vi "PIV_Stats.vi"(0 "Data Folder":path=path "T:/Ensight_Data/NACA0015/NACA0015_NM_B/Test_A", 1 "PIV Meas Plane":enum16{"XY", "YZ", "XZ"}(ring)=enum."XZ", 2 "Row number":i32=1, 5 "Output Directory":path=path "T:/Ensight_Data/NACA0015/NACA0015_NM_B", 7 "XYZ Translation":dbl[](array[numeric])=[200.0, 8.0, -30.0], 9 "Case Name":string="Test_A_Case", 11 "PIV Freq (Hz)":dbl=7.25, 12 "Invert U":bool=TRUE, 13 "Invert V":bool) -> (4 "Progress Bar":i32(slide) scale=0.0..100.0, 6 "Status":string, 10 "# total vectors":i32=9858, 15 "# vectors without records":i16)   [LabVIEW 2011]
uses:
  <vilib>/Utility/error.llb/DialogType.ctl
  <vilib>/Analysis/1siggen.llb/Ramp Pattern by Samples.vi
  <vilib>/Analysis/NI_AALBase.lvlib
panel:
  out "VectRawData(time,spot)":dbl[][][](array[numeric])
  out "Position Array":dbl[][](array[numeric])
  out "Data Array":dbl[][][](array[numeric])
  out "Tmax":dbl=0.41379310344827586
  out "Max Record Length":i32=3
  out "Variable Names":string[](array[string])=["Record_Length", "CHC", "u_ms", "v_ms", "time_s", "Vel_mag_ms", "Turb_Stats_U_ms", "Turb_Stats_u2_m2s2", "Turb_Stats_u3_m3s3", "Turb_Stats_u4_m4s4", "Turb_Stats_TurbU_%", "Turb_Stats_Skew_u", "Turb_Stats_Kurt_u", "Turb_Stats_V_ms", "Turb_Stats_v2_m2s2", "Turb_Stats_v3_m3s3", "Turb_Stats_v4_m4s4", "Turb_Stats_TurbV_%", "Turb_Stats_Skew_v", "Turb_Stats_Kurt_v", "Turb_Stats_u2v2_m4s4", "Turb_Stats_uv3_m4s4", "Turb_Stats_u3v_m4s4", "Turb_Stats_uv2_m3s3", "Turb_Stats_u2v_m3s3", "Turb_Stats_uv_cc", "Turb_Stats_uv", "Turb_Stats_TKE_J", "Turb_Stats_Error_U_ms", "Turb_Stats_Error_u2_m2s2", "Turb_Stats_Error_u3_m3s3", "Turb_Stats_Error_u4_m4s4", "Turb_Stats_Error_TurbU_%", "Turb_Stats_Error_Skew_u", "Turb_Stats_Error_Kurt_u", "Turb_Stats_Error_V_ms", "Turb_Stats_Error_v2_m2s2", "Turb_Stats_Error_v3_m3s3", "Turb_Stats_Error_v4_m4s4", "Turb_Stats_Error_TurbV_%", "Turb_Stats_Error_Skew_v", "Turb_Stats_Error_Kurt_v", "Turb_Stats_Error_u2v2_m4s4", "Turb_Stats_Error_uv3_m4s4", "Turb_Stats_Error_u3v_m4s4", "Turb_Stats_Error_uv2_m3s3", "Turb_Stats_Error_u2v_m3s3", "Turb_Stats_Error_uv_cc", "Turb_Stats_Error_uv", "Turb_Stats_Error_TKE_J"]
  out "File Paths":path[][](array[path])=[[path "C:/Users/Nick/Desktop/Test/Testing/ENSI_0000.case", path "C:/Users/Nick/Desktop/Test/Testing/ENSI_0000.geo", path "C:/Users/Nick/Desktop/Test/Testing/ENSI_0000.var1", path "C:/Users/Nick/Desktop/Test/Testing/ENSI_0000.var2", path "C:/Users/Nick/Desktop/Test/Testing/ENSI_0000.var3", path "C:/Users/Nick/Desktop/Test/Testing/ENSI_0000.var4", path "C:/Users/Nick/Desktop/Test/Testing/ENSI_0000.var5", path "C:/Users/Nick/Desktop/Test/Testing/ENSI_0000.var6", path "C:/Users/Nick/Desktop/Test/Testing/ENSI_0000.var7", path "C:/Users/Nick/Desktop/Test/Testing/ENSI_0000.var8", path "C:/Users/Nick/Desktop/Test/Testing/ENSI_0000.var9", path "C:/Users/Nick/Desktop/Test/Testing/ENSI_0000.var10", path "C:/Users/Nick/Desktop/Test/Testing/ENSI_0000.var11", path "C:/Users/Nick/Desktop/Test/Testing/ENSI_0000.var12", path "C:/Users/Nick/Desktop/Test/Testing/ENSI_0000.var13", path "C:/Users/Nick/Desktop/Test/Testing/ENSI_0000.var14", path "C:/Users/Nick/Desktop/Test/Testing/ENSI_0000.var15", path "C:/Users/Nick/Desktop/Test/Testing/ENSI_0000.var16", path "C:/Users/Nick/Desktop/Test/Testing/ENSI_0000.var17", path "C:/Users/Nick/Desktop/Test/Testing/ENSI_0000.var18", path "C:/Users/Nick/Desktop/Test/Testing/ENSI_0000.var19", path "C:/Users/Nick/Desktop/Test/Testing/ENSI_0000.var20", path "C:/Users/Nick/Desktop/Test/Testing/ENSI_0000.var21", path "C:/Users/Nick/Desktop/Test/Testing/ENSI_0000.var22", path "C:/Users/Nick/Desktop/Test/Testing/ENSI_0000.var23", path "C:/Users/Nick/Desktop/Test/Testing/ENSI_0000.var24", path "C:/Users/Nick/Desktop/Test/Testing/ENSI_0000.var25", path "C:/Users/Nick/Desktop/Test/Testing/ENSI_0000.var26", path "C:/Users/Nick/Desktop/Test/Testing/ENSI_0000.var27", path "C:/Users/Nick/Desktop/Test/Testing/ENSI_0000.var28", path "C:/Users/Nick/Desktop/Test/Testing/ENSI_0000.var29", path "C:/Users/Nick/Desktop/Test/Testing/ENSI_0000.var30", path "C:/Users/Nick/Desktop/Test/Testing/ENSI_0000.var31", path "C:/Users/Nick/Desktop/Test/Testing/ENSI_0000.var32", path "C:/Users/Nick/Desktop/Test/Testing/ENSI_0000.var33", path "C:/Users/Nick/Desktop/Test/Testing/ENSI_0000.var34", path "C:/Users/Nick/Desktop/Test/Testing/ENSI_0000.var35", path "C:/Users/Nick/Desktop/Test/Testing/ENSI_0000.var36", path "C:/Users/Nick/Desktop/Test/Testing/ENSI_0000.var37", path "C:/Users/Nick/Desktop/Test/Testing/ENSI_0000.var38", path "C:/Users/Nick/Desktop/Test/Testing/ENSI_0000.var39", path "C:/Users/Nick/Desktop/Test/Testing/ENSI_0000.var40", path "C:/Users/Nick/Desktop/Test/Testing/ENSI_0000.var41", path "C:/Users/Nick/Desktop/Test/Testing/ENSI_0000.var42", path "C:/Users/Nick/Desktop/Test/Testing/ENSI_0000.var43", path "C:/Users/Nick/Desktop/Test/Testing/ENSI_0000.var44", path "C:/Users/Nick/Desktop/Test/Testing/ENSI_0000.var45", path "C:/Users/Nick/Desktop/Test/Testing/ENSI_0000.var46", path "C:/Users/Nick/Desktop/Test/Testing/ENSI_0000.var47", path "C:/Users/Nick/Desktop/Test/Testing/ENSI_0000.var48", path "C:/Users/Nick/Desktop/Test/Testing/ENSI_0000.var49", path "C:/Users/Nick/Desktop/Test/Testing/ENSI_0000.var50"], [path "C:/Users/Nick/Desktop/Test/Testing/ENSI_0001.case", path "C:/Users/Nick/Desktop/Test/Testing/ENSI_0001.geo", path "C:/Users/Nick/Desktop/Test/Testing/ENSI_0001.var1", path "C:/Users/Nick/Desktop/Test/Testing/ENSI_0001.var2", path "C:/Users/Nick/Desktop/Test/Testing/ENSI_0001.var3", path "C:/Users/Nick/Desktop/Test/Testing/ENSI_0001.var4", path "C:/Users/Nick/Desktop/Test/Testing/ENSI_0001.var5", path "C:/Users/Nick/Desktop/Test/Testing/ENSI_0001.var6", path "C:/Users/Nick/Desktop/Test/Testing/ENSI_0001.var7", path "C:/Users/Nick/Desktop/Test/Testing/ENSI_0001.var8", path "C:/Users/Nick/Desktop/Test/Testing/ENSI_0001.var9", path "C:/Users/Nick/Desktop/Test/Testing/ENSI_0001.var10", path "C:/Users/Nick/Desktop/Test/Testing/ENSI_0001.var11", path "C:/Users/Nick/Desktop/Test/Testing/ENSI_0001.var12", path "C:/Users/Nick/Desktop/Test/Testing/ENSI_0001.var13", path "C:/Users/Nick/Desktop/Test/Testing/ENSI_0001.var14", path "C:/Users/Nick/Desktop/Test/Testing/ENSI_0001.var15", path "C:/Users/Nick/Desktop/Test/Testing/ENSI_0001.var16", path "C:/Users/Nick/Desktop/Test/Testing/ENSI_0001.var17", path "C:/Users/Nick/Desktop/Test/Testing/ENSI_0001.var18", path "C:/Users/Nick/Desktop/Test/Testing/ENSI_0001.var19", path "C:/Users/Nick/Desktop/Test/Testing/ENSI_0001.var20", path "C:/Users/Nick/Desktop/Test/Testing/ENSI_0001.var21", path "C:/Users/Nick/Desktop/Test/Testing/ENSI_0001.var22", path "C:/Users/Nick/Desktop/Test/Testing/ENSI_0001.var23", path "C:/Users/Nick/Desktop/Test/Testing/ENSI_0001.var24", path "C:/Users/Nick/Desktop/Test/Testing/ENSI_0001.var25", path "C:/Users/Nick/Desktop/Test/Testing/ENSI_0001.var26", path "C:/Users/Nick/Desktop/Test/Testing/ENSI_0001.var27", path "C:/Users/Nick/Desktop/Test/Testing/ENSI_0001.var28", path "C:/Users/Nick/Desktop/Test/Testing/ENSI_0001.var29", path "C:/Users/Nick/Desktop/Test/Testing/ENSI_0001.var30", path "C:/Users/Nick/Desktop/Test/Testing/ENSI_0001.var31", path "C:/Users/Nick/Desktop/Test/Testing/ENSI_0001.var32", path "C:/Users/Nick/Desktop/Test/Testing/ENSI_0001.var33", path "C:/Users/Nick/Desktop/Test/Testing/ENSI_0001.var34", path "C:/Users/Nick/Desktop/Test/Testing/ENSI_0001.var35", path "C:/Users/Nick/Desktop/Test/Testing/ENSI_0001.var36", path "C:/Users/Nick/Desktop/Test/Testing/ENSI_0001.var37", path "C:/Users/Nick/Desktop/Test/Testing/ENSI_0001.var38", path "C:/Users/Nick/Desktop/Test/Testing/ENSI_0001.var39", path "C:/Users/Nick/Desktop/Test/Testing/ENSI_0001.var40", path "C:/Users/Nick/Desktop/Test/Testing/ENSI_0001.var41", path "C:/Users/Nick/Desktop/Test/Testing/ENSI_0001.var42", path "C:/Users/Nick/Desktop/Test/Testing/ENSI_0001.var43", path "C:/Users/Nick/Desktop/Test/Testing/ENSI_0001.var44", path "C:/Users/Nick/Desktop/Test/Testing/ENSI_0001.var45", path "C:/Users/Nick/Desktop/Test/Testing/ENSI_0001.var46", path "C:/Users/Nick/Desktop/Test/Testing/ENSI_0001.var47", path "C:/Users/Nick/Desktop/Test/Testing/ENSI_0001.var48", path "C:/Users/Nick/Desktop/Test/Testing/ENSI_0001.var49", path "C:/Users/Nick/Desktop/Test/Testing/ENSI_0001.var50"], [path "C:/Users/Nick/Desktop/Test/Testing/ENSI_0002.case", path "C:/Users/Nick/Desktop/Test/Testing/ENSI_0002.geo", path "C:/Users/Nick/Desktop/Test/Testing/ENSI_0002.var1", path "C:/Users/Nick/Desktop/Test/Testing/ENSI_0002.var2", path "C:/Users/Nick/Desktop/Test/Testing/ENSI_0002.var3", path "C:/Users/Nick/Desktop/Test/Testing/ENSI_0002.var4", path "C:/Users/Nick/Desktop/Test/Testing/ENSI_0002.var5", path "C:/Users/Nick/Desktop/Test/Testing/ENSI_0002.var6", path "C:/Users/Nick/Desktop/Test/Testing/ENSI_0002.var7", path "C:/Users/Nick/Desktop/Test/Testing/ENSI_0002.var8", path "C:/Users/Nick/Desktop/Test/Testing/ENSI_0002.var9", path "C:/Users/Nick/Desktop/Test/Testing/ENSI_0002.var10", path "C:/Users/Nick/Desktop/Test/Testing/ENSI_0002.var11", path "C:/Users/Nick/Desktop/Test/Testing/ENSI_0002.var12", path "C:/Users/Nick/Desktop/Test/Testing/ENSI_0002.var13", path "C:/Users/Nick/Desktop/Test/Testing/ENSI_0002.var14", path "C:/Users/Nick/Desktop/Test/Testing/ENSI_0002.var15", path "C:/Users/Nick/Desktop/Test/Testing/ENSI_0002.var16", path "C:/Users/Nick/Desktop/Test/Testing/ENSI_0002.var17", path "C:/Users/Nick/Desktop/Test/Testing/ENSI_0002.var18", path "C:/Users/Nick/Desktop/Test/Testing/ENSI_0002.var19", path "C:/Users/Nick/Desktop/Test/Testing/ENSI_0002.var20", path "C:/Users/Nick/Desktop/Test/Testing/ENSI_0002.var21", path "C:/Users/Nick/Desktop/Test/Testing/ENSI_0002.var22", path "C:/Users/Nick/Desktop/Test/Testing/ENSI_0002.var23", path "C:/Users/Nick/Desktop/Test/Testing/ENSI_0002.var24", path "C:/Users/Nick/Desktop/Test/Testing/ENSI_0002.var25", path "C:/Users/Nick/Desktop/Test/Testing/ENSI_0002.var26", path "C:/Users/Nick/Desktop/Test/Testing/ENSI_0002.var27", path "C:/Users/Nick/Desktop/Test/Testing/ENSI_0002.var28", path "C:/Users/Nick/Desktop/Test/Testing/ENSI_0002.var29", path "C:/Users/Nick/Desktop/Test/Testing/ENSI_0002.var30", path "C:/Users/Nick/Desktop/Test/Testing/ENSI_0002.var31", path "C:/Users/Nick/Desktop/Test/Testing/ENSI_0002.var32", path "C:/Users/Nick/Desktop/Test/Testing/ENSI_0002.var33", path "C:/Users/Nick/Desktop/Test/Testing/ENSI_0002.var34", path "C:/Users/Nick/Desktop/Test/Testing/ENSI_0002.var35", path "C:/Users/Nick/Desktop/Test/Testing/ENSI_0002.var36", path "C:/Users/Nick/Desktop/Test/Testing/ENSI_0002.var37", path "C:/Users/Nick/Desktop/Test/Testing/ENSI_0002.var38", path "C:/Users/Nick/Desktop/Test/Testing/ENSI_0002.var39", path "C:/Users/Nick/Desktop/Test/Testing/ENSI_0002.var40", path "C:/Users/Nick/Desktop/Test/Testing/ENSI_0002.var41", path "C:/Users/Nick/Desktop/Test/Testing/ENSI_0002.var42", path "C:/Users/Nick/Desktop/Test/Testing/ENSI_0002.var43", path "C:/Users/Nick/Desktop/Test/Testing/ENSI_0002.var44", path "C:/Users/Nick/Desktop/Test/Testing/ENSI_0002.var45", path "C:/Users/Nick/Desktop/Test/Testing/ENSI_0002.var46", path "C:/Users/Nick/Desktop/Test/Testing/ENSI_0002.var47", path "C:/Users/Nick/Desktop/Test/Testing/ENSI_0002.var48", path "C:/Users/Nick/Desktop/Test/Testing/ENSI_0002.var49", path "C:/Users/Nick/Desktop/Test/Testing/ENSI_0002.var50"]]
  out "ALL filepath":path=path "C:/Users/Nick/Desktop/Test/Testing/ENSI_all.case"
  out "time s":dbl[](array[numeric])=[0.0, 0.20689655172413793, 0.41379310344827586]
  out "File Array":path[](array[path])=[path "T:/Ensight_Data/NACA0015/NACA0015_NM_A/Test_A_Trans/New folder/Test_A000000.T076.D000.P000.H000.L.vec", path "T:/Ensight_Data/NACA0015/NACA0015_NM_A/Test_A_Trans/New folder/Test_A000001.T076.D000.P000.H000.L.vec", path "T:/Ensight_Data/NACA0015/NACA0015_NM_A/Test_A_Trans/New folder/Test_A000002.T076.D000.P000.H000.L.vec"]
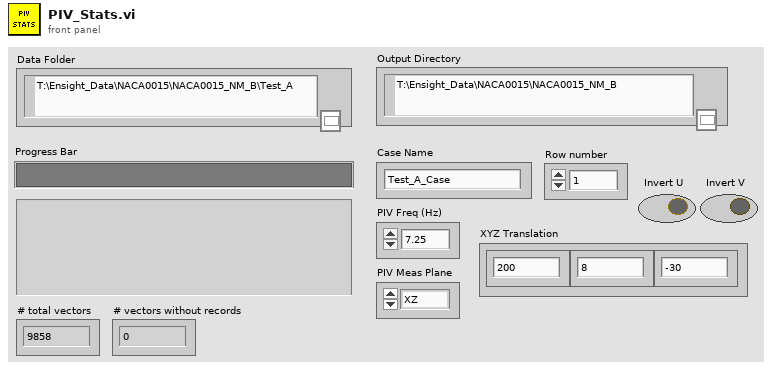
[diagram p1: front panel]
types:
  T1 = cluster{"Record Length":dbl, "CHC":dbl[], "u m/s":dbl[], "v m/s":dbl[], "time s":dbl[], "Vel mag m/s":dbl[], "XYZ Position":dbl[], " Turb Stats":cluster{"U m/s":dbl, "u2 m2/s2":dbl, "u3 m3/s3":dbl, "u4 m4/s4":dbl, "TurbU %":dbl, "Skew_u":dbl, "Kurt_u":dbl, "V m/s":dbl, "v2 m2/s2":dbl, "v3 m3/s3":dbl, "v4 m4/s4":dbl, "TurbV %":dbl, "Skew_v":dbl, "Kurt_v":dbl, "u2v2 m4/s4":dbl, "uv3 m4/s4":dbl, "u3v m4/s4":dbl, "uv2 m3/s3":dbl, "u2v m3/s3":dbl, "uv_cc":dbl, "uv":dbl, "TKE J":dbl}[], "Turb Stats Error":cluster{"U m/s":dbl, "u2 m2/s2":dbl, "u3 m3/s3":dbl, "u4 m4/s4":dbl, "TurbU %":dbl, "Skew_u":dbl, "Kurt_u":dbl, "V m/s":dbl, "v2 m2/s2":dbl, "v3 m3/s3":dbl, "v4 m4/s4":dbl, "TurbV %":dbl, "Skew_v":dbl, "Kurt_v":dbl, "u2v2 m4/s4":dbl, "uv3 m4/s4":dbl, "u3v m4/s4":dbl, "uv2 m3/s3":dbl, "u2v m3/s3":dbl, "uv_cc":dbl, "uv":dbl, "TKE J":dbl}[], "u (good)":dbl[], "v (good)":dbl[]}
  T2 = cluster{"Record Length":dbl, "CHC":dbl[], "u m/s":dbl[], "v m/s":dbl[], "time s":dbl[], "Vel mag m/s":dbl[], "XYZ Position":dbl[], " Turb Stats":cluster{"U m/s":dbl, "u2 m2/s2":dbl, "u3 m3/s3":dbl, "u4 m4/s4":dbl, "TurbU %":dbl, "Skew_u":dbl, "Kurt_u":dbl, "V m/s":dbl, "v2 m2/s2":dbl, "v3 m3/s3":dbl, "v4 m4/s4":dbl, "TurbV %":dbl, "Skew_v":dbl, "Kurt_v":dbl, "u2v2 m4/s4":dbl, "uv3 m4/s4":dbl, "u3v m4/s4":dbl, "uv2 m3/s3":dbl, "u2v m3/s3":dbl, "uv_cc":dbl, "uv":dbl, "TKE J":dbl}[], "Turb Stats Error":cluster{"U m/s":dbl, "u2 m2/s2":dbl, "u3 m3/s3":dbl, "u4 m4/s4":dbl, "TurbU %":dbl, "Skew_u":dbl, "Kurt_u":dbl, "V m/s":dbl, "v2 m2/s2":dbl, "v3 m3/s3":dbl, "v4 m4/s4":dbl, "TurbV %":dbl, "Skew_v":dbl, "Kurt_v":dbl, "u2v2 m4/s4":dbl, "uv3 m4/s4":dbl, "u3v m4/s4":dbl, "uv2 m3/s3":dbl, "u2v m3/s3":dbl, "uv_cc":dbl, "uv":dbl, "TKE J":dbl}[], "u (good)":dbl[], "v (good)":dbl[]}[]
  T3 = cluster{"U m/s":dbl, "u2 m2/s2":dbl, "u3 m3/s3":dbl, "u4 m4/s4":dbl, "TurbU %":dbl, "Skew_u":dbl, "Kurt_u":dbl, "V m/s":dbl, "v2 m2/s2":dbl, "v3 m3/s3":dbl, "v4 m4/s4":dbl, "TurbV %":dbl, "Skew_v":dbl, "Kurt_v":dbl, "u2v2 m4/s4":dbl, "uv3 m4/s4":dbl, "u3v m4/s4":dbl, "uv2 m3/s3":dbl, "u2v m3/s3":dbl, "uv_cc":dbl, "uv":dbl, "TKE J":dbl}
  T4 = cluster{"U m/s":dbl, "u2 m2/s2":dbl, "u3 m3/s3":dbl, "u4 m4/s4":dbl, "TurbU %":dbl, "Skew_u":dbl, "Kurt_u":dbl, "V m/s":dbl, "v2 m2/s2":dbl, "v3 m3/s3":dbl, "v4 m4/s4":dbl, "TurbV %":dbl, "Skew_v":dbl, "Kurt_v":dbl, "u2v2 m4/s4":dbl, "uv3 m4/s4":dbl, "u3v m4/s4":dbl, "uv2 m3/s3":dbl, "u2v m3/s3":dbl, "uv_cc":dbl, "uv":dbl, "TKE J":dbl}[]
  T5 = typedef "DialogType.ctl" = u16
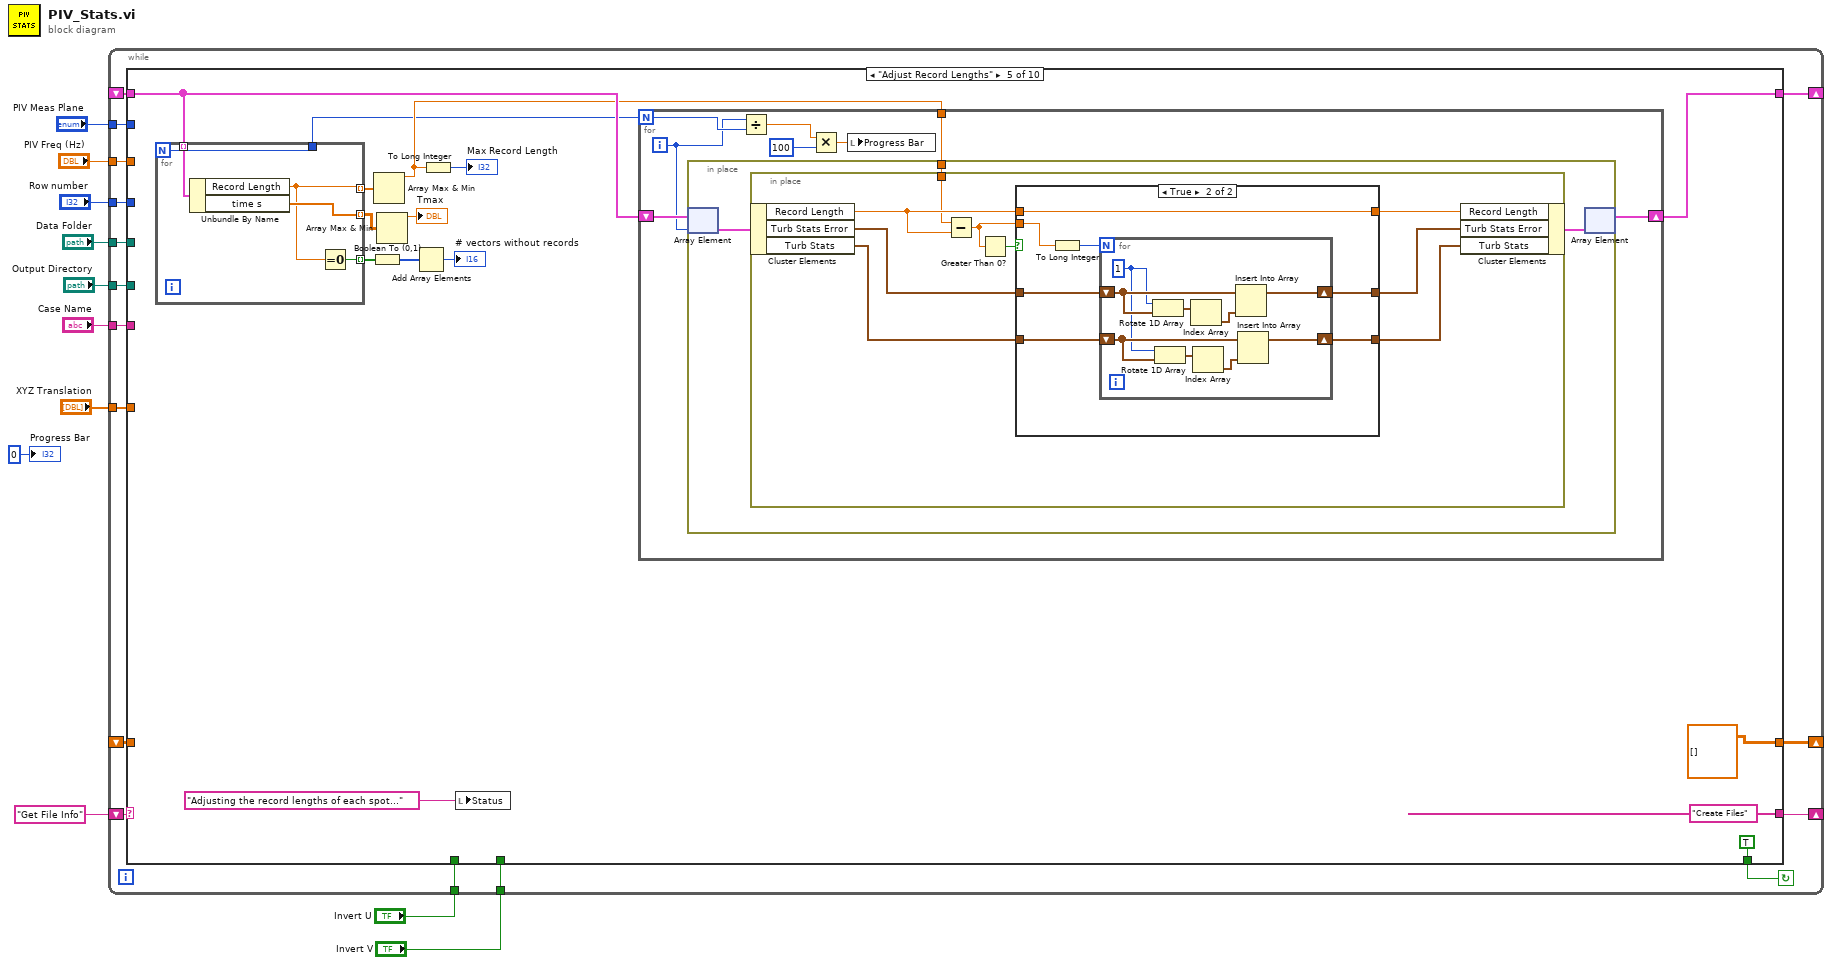
[diagram p0: block diagram]
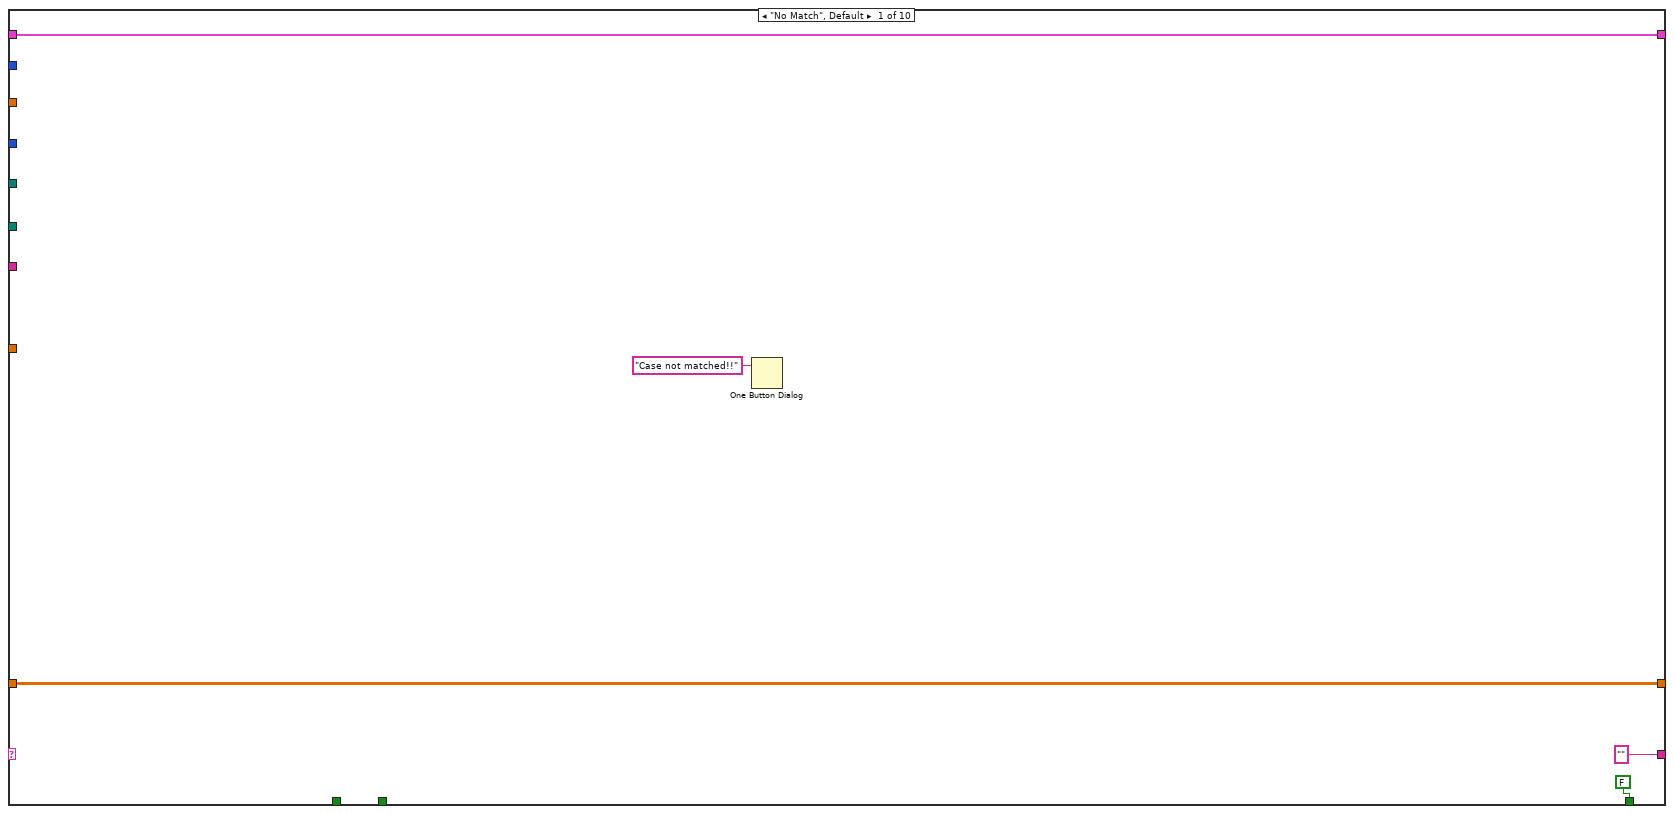
[diagram p2: hidden frame]
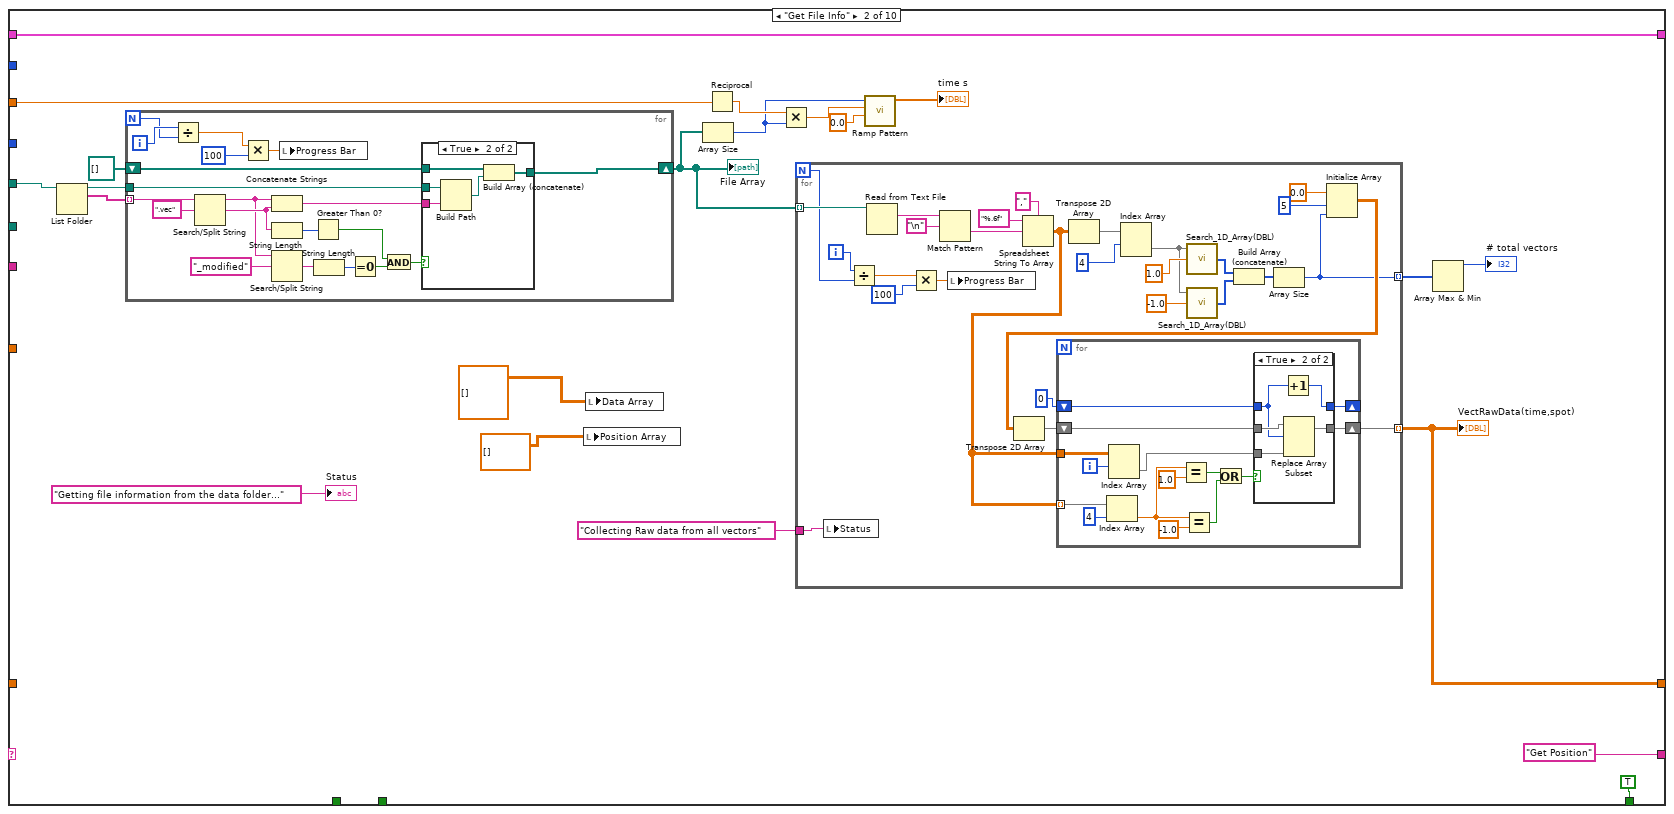
[diagram p3: hidden frame]
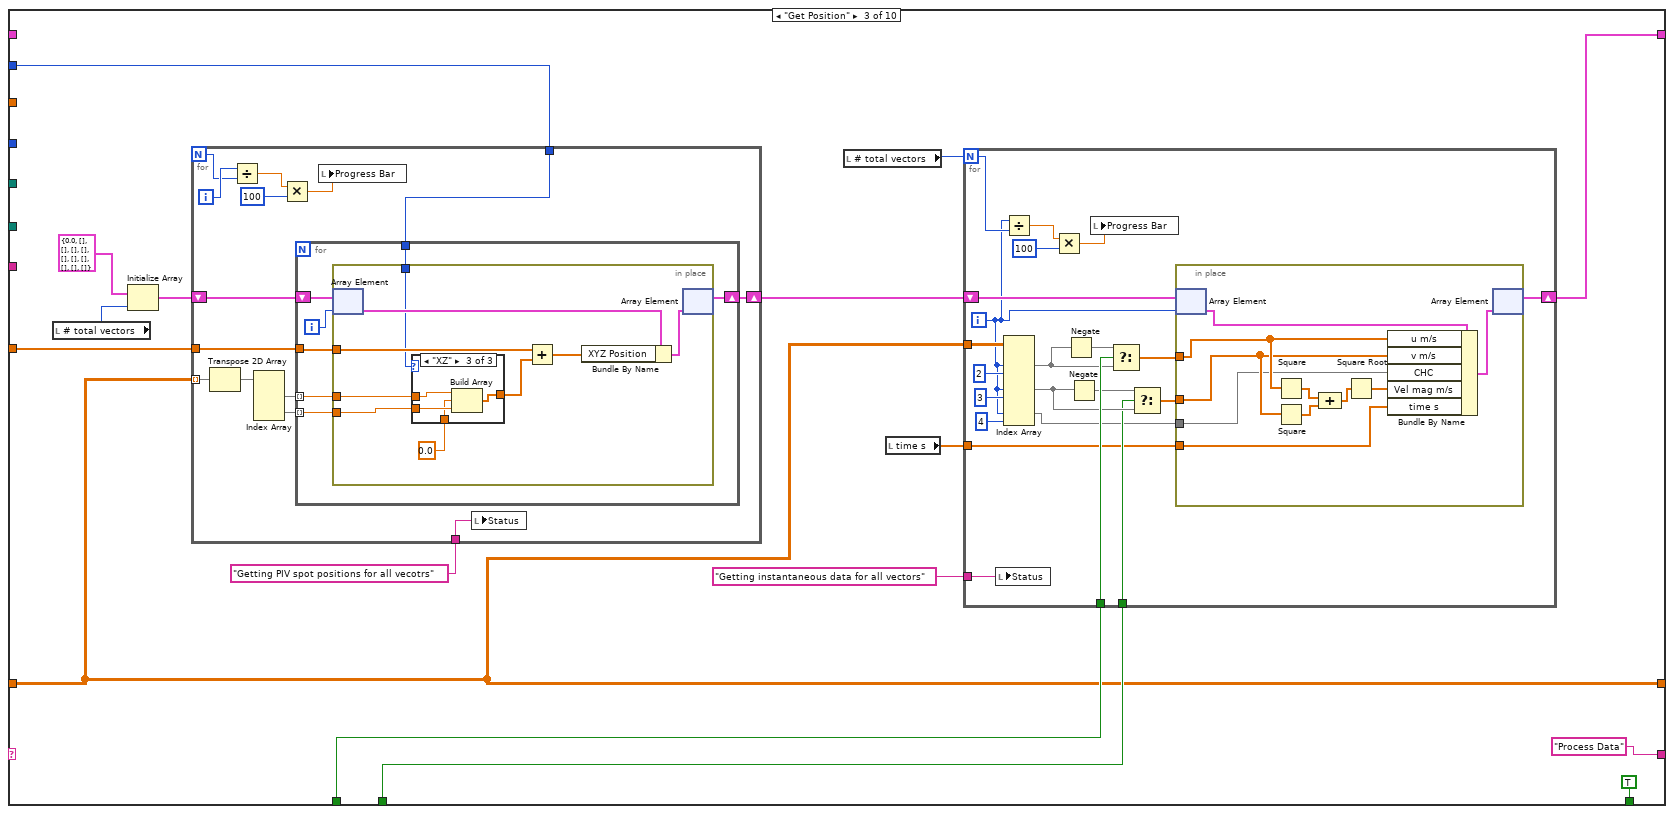
[diagram p6: hidden frame]
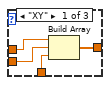
[diagram p7: hidden frame]
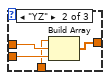
[diagram p8: hidden frame]
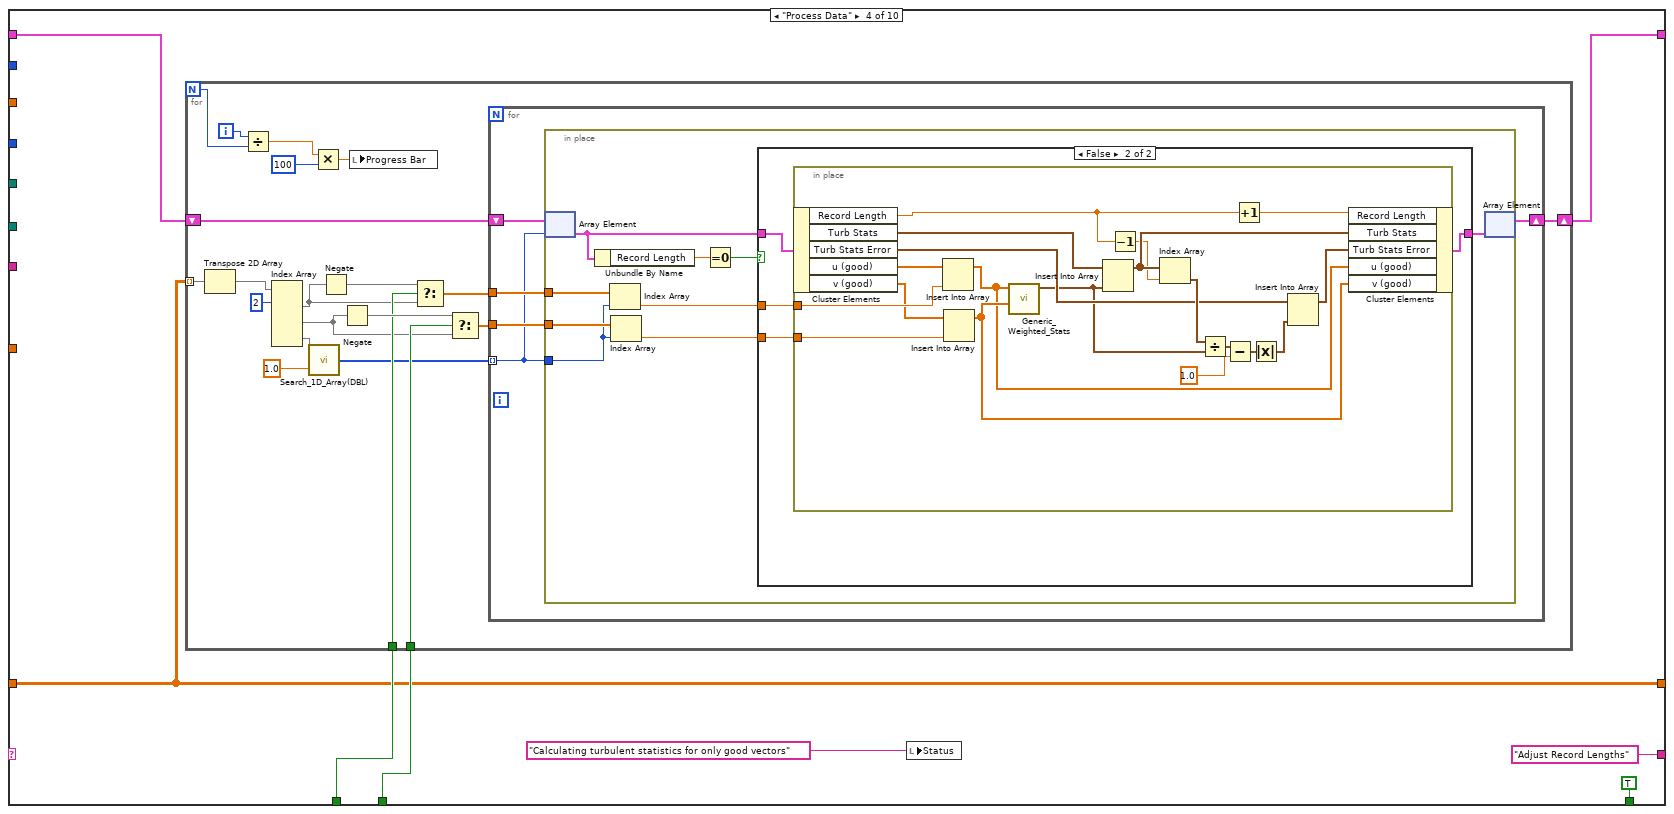
[diagram p9: hidden frame]
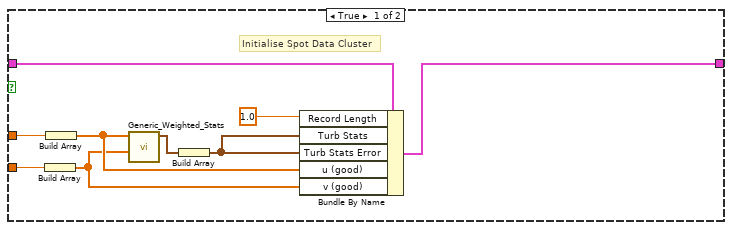
[diagram p10: hidden frame]
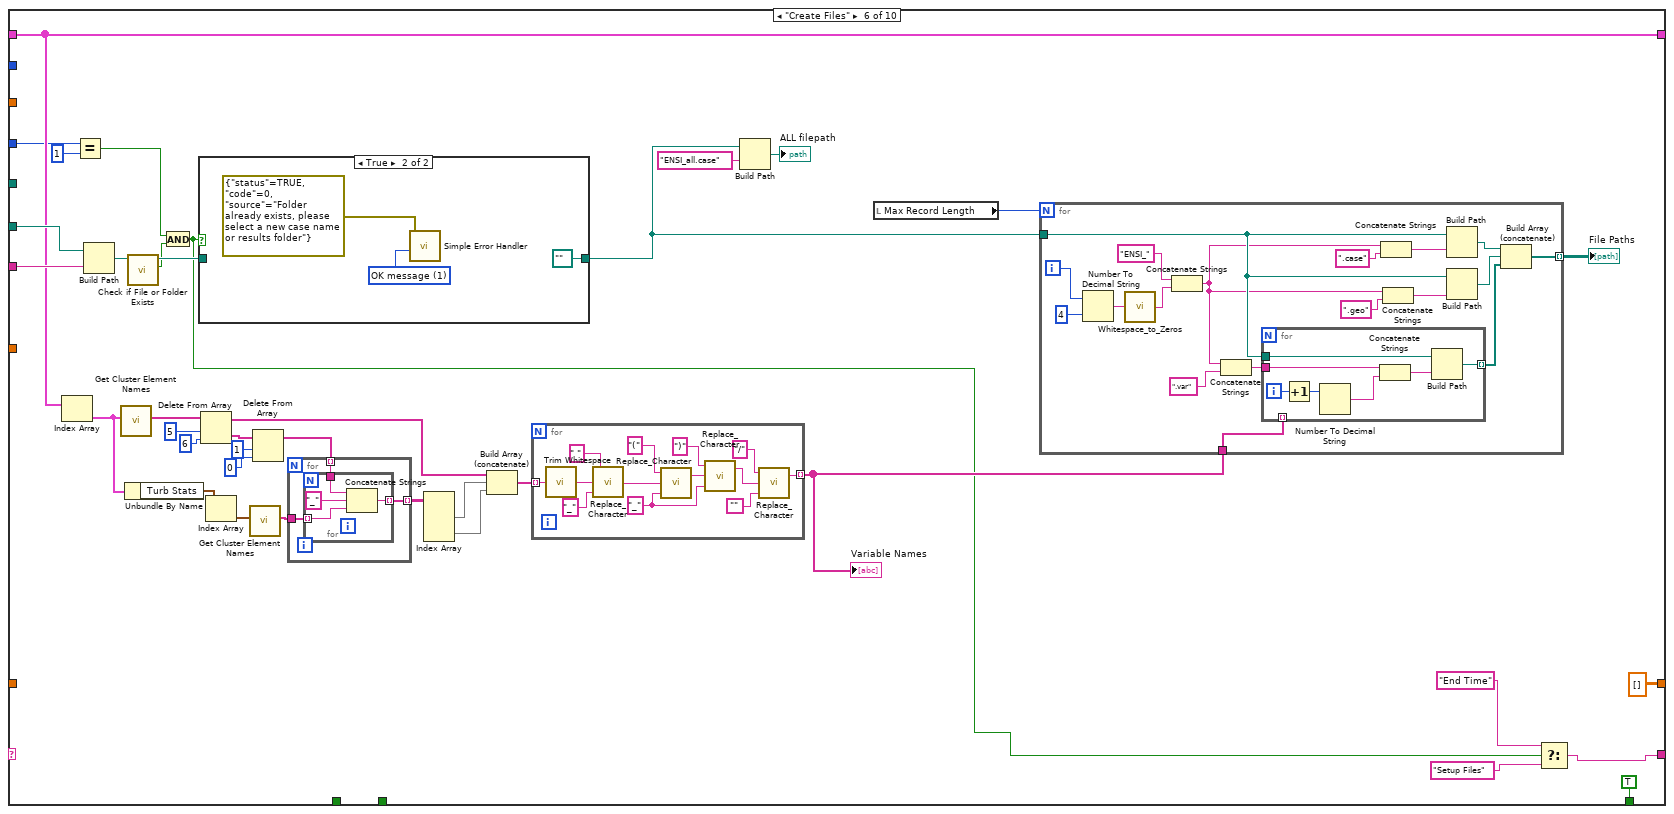
[diagram p12: hidden frame]
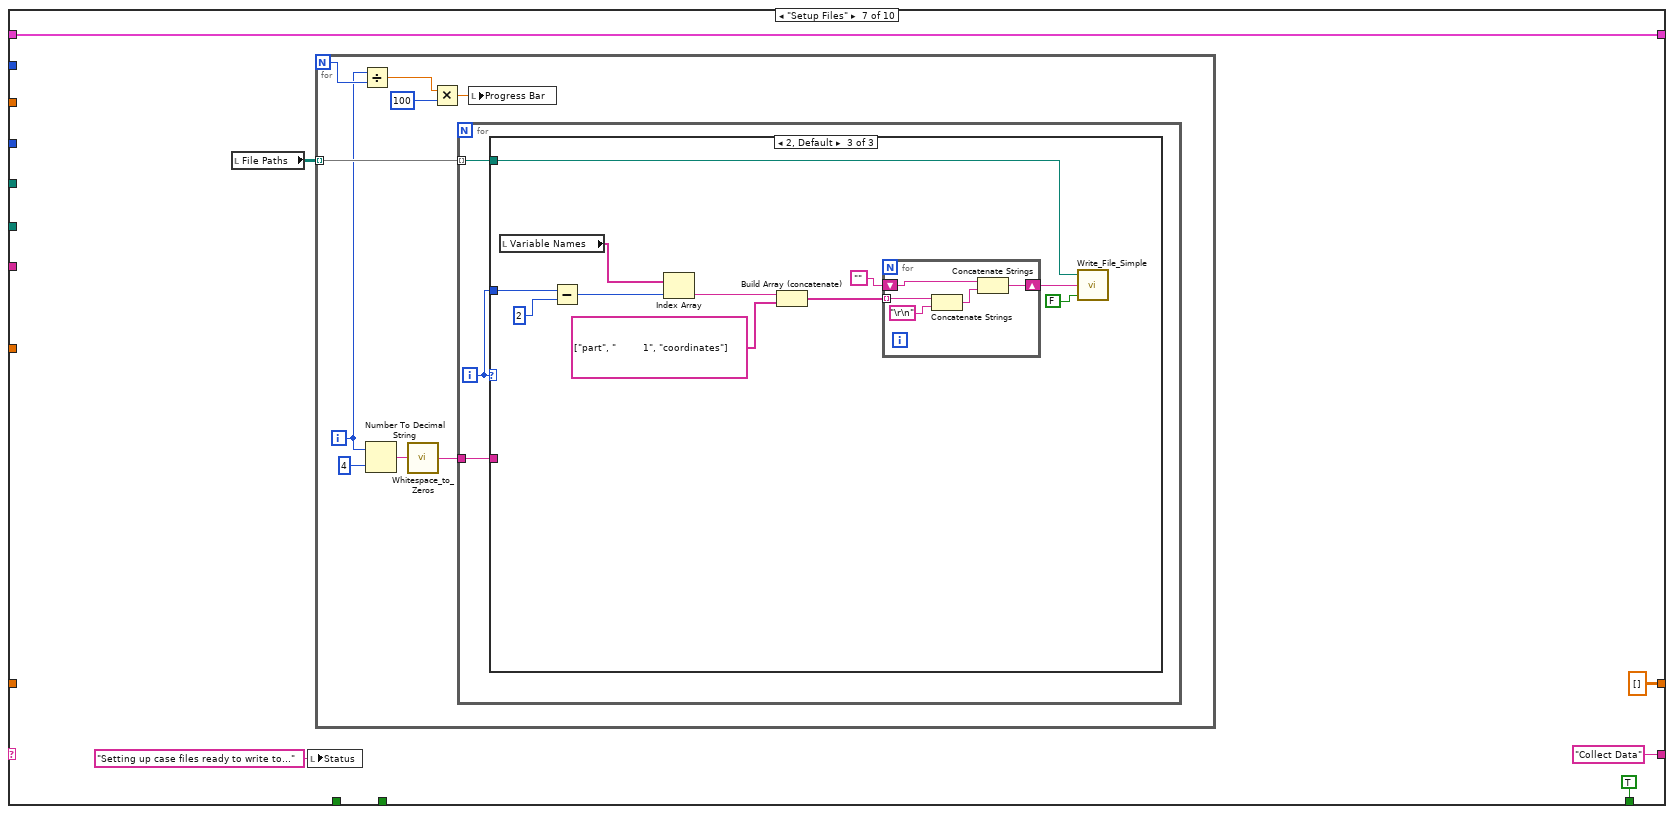
[diagram p14: hidden frame]
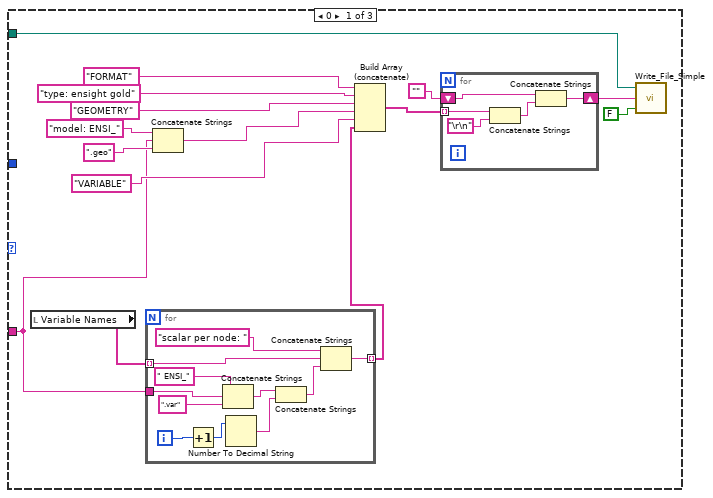
[diagram p15: hidden frame]
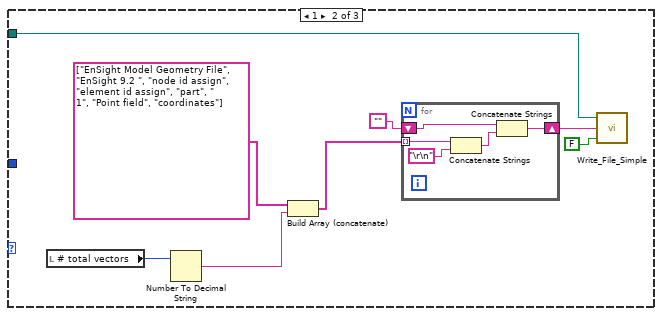
[diagram p16: hidden frame]
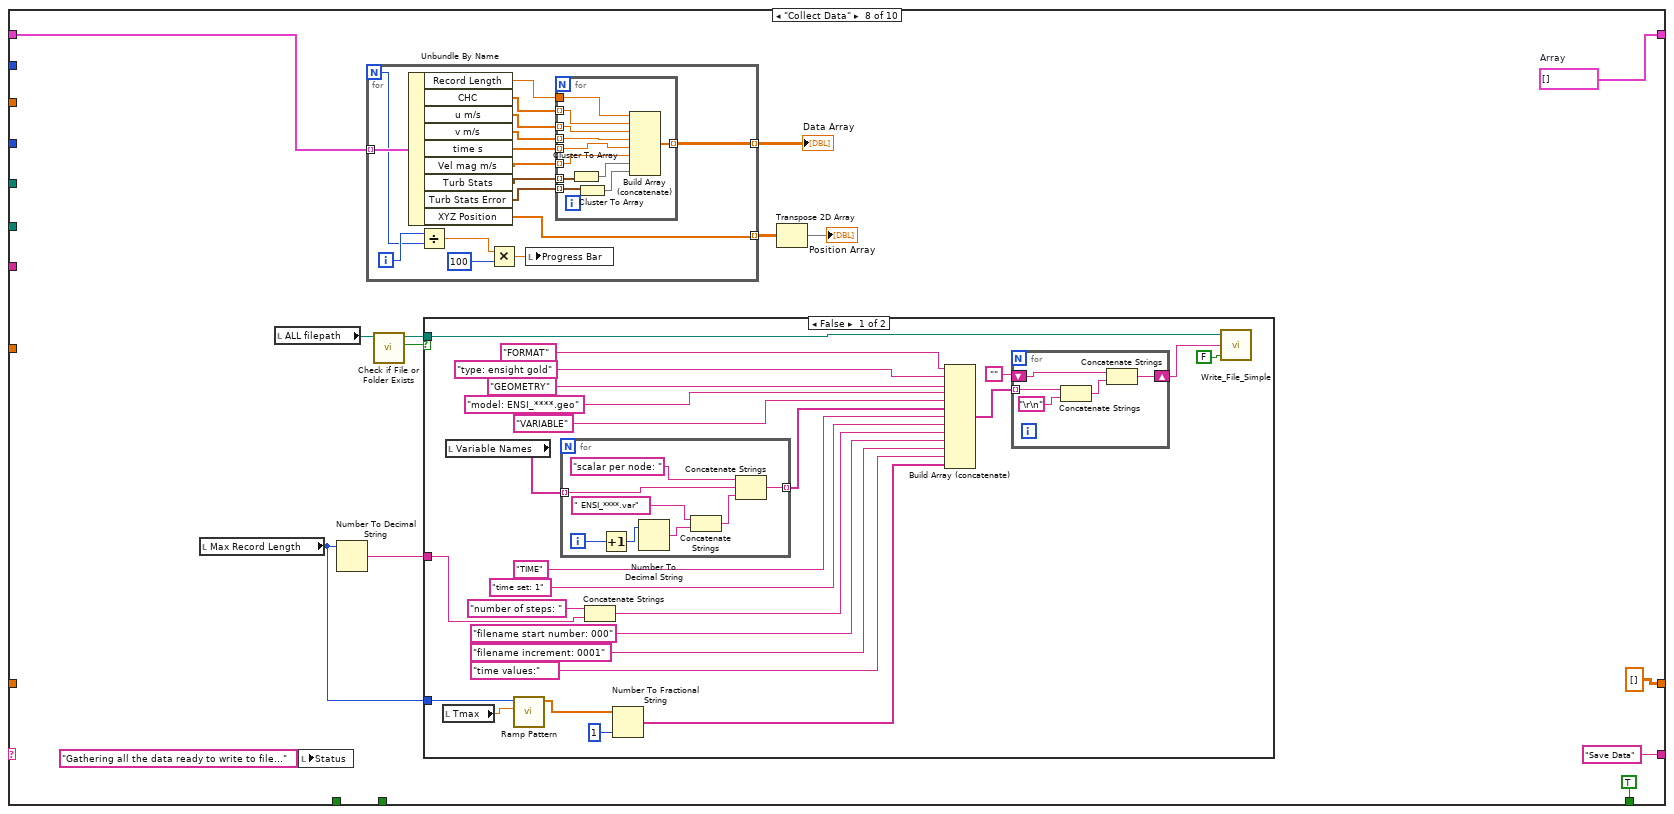
[diagram p17: hidden frame]
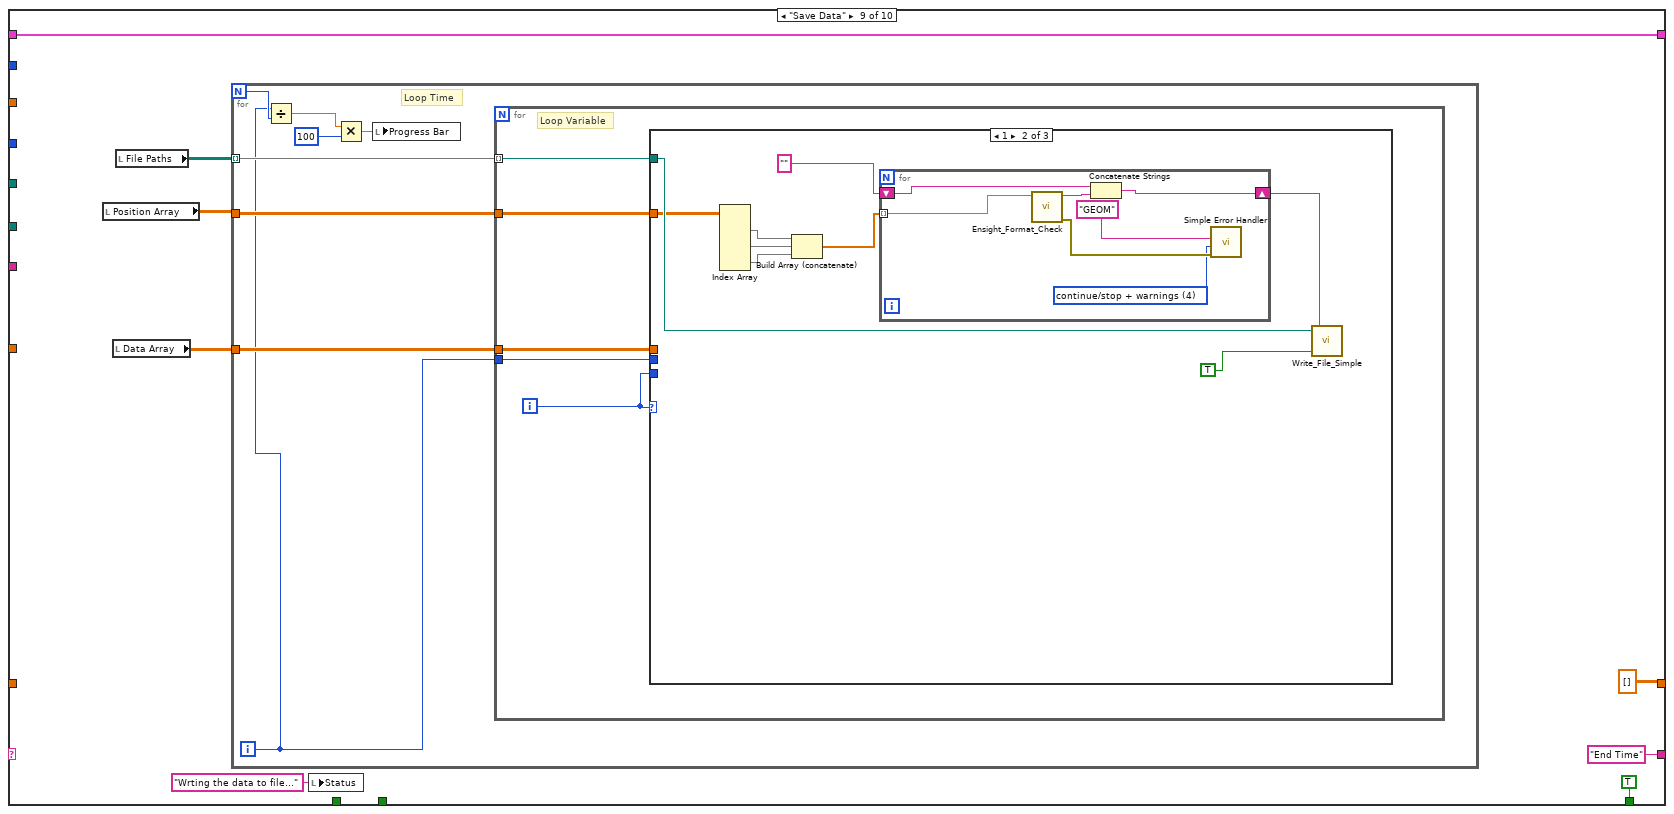
[diagram p19: hidden frame]
diagram:
  n1 = while {
    shift-right: [w26] -> _
    shift-left: "Get File Info" -> [w27]
    tunnel: "Data Folder" -> [w25]
    tunnel: "Output Directory" -> [w23]
    tunnel: "Case Name" -> [w22]
    tunnel: "PIV Freq (Hz)" -> [w21]
    tunnel: "PIV Meas Plane" -> [w20]
    tunnel: "XYZ Translation" -> [w19]
    shift-right: [w18] -> _
    shift-left: _ -> [w17]
    tunnel: "Row number" -> [w16]
    tunnel: "Invert V" -> [w15]
    tunnel: "Invert U" -> [w14]
    shift-right: [w13] -> _
    shift-left: _ -> [w12]
    stop <- w24 continue-if-true
    n2 = case shown="\"Adjust Record Lengths\"" w27 {
      tunnel: ["" "Get Position" "Process Data" "Adjust Record Lengths" "Create Files" w358 "Collect Data" ("t") "Save Data" ("t") "End Time" ("t") "" ("t")] -> w26
      tunnel: w25 -> [_ w48 _ _ _ _ _ _ _ _]
      tunnel: [FALSE TRUE TRUE TRUE TRUE TRUE TRUE TRUE TRUE FALSE] -> w24
      tunnel: w23 -> [_ _ _ _ _ w386 _ _ _ _]
      tunnel: w22 -> [_ _ _ _ _ w387 _ _ _ _]
      tunnel: w21 -> [_ w47 _ _ _ _ _ _ _ _]
      tunnel: w20 -> [_ _ w142 _ _ _ _ _ _ _]
      tunnel: w19 -> [_ _ w143 _ _ _ _ _ _ _]
      tunnel: [w30 w35 w134 w225 w307 w370 w442 w519 w602 w655] -> w18
      tunnel: w17 -> [w30 w35 _ w223 w306 w370 w442 w524 w602 w655]
      tunnel: w16 -> [_ _ _ _ _ w365 _ _ _ _]
      tunnel: w15 -> [_ _ w133 w222 _ _ _ _ _ _]
      tunnel: w14 -> [_ _ w132 w221 _ _ _ _ _ _]
      tunnel: [w28 w33 w130 w220 dbl[][][] [] ("GoodRawData(time,spot)") dbl[][][] [] ("GoodRawData(time,spot)") dbl[][][] [] ("GoodRawData(time,spot)") dbl[][][] [] ("GoodRawData(time,spot)") dbl[][][] [] ("GoodRawData(time,spot)") w654] -> w13
      tunnel: w12 -> [w28 _ w130 w220 _ _ _ _ _ w654]
      frame "No Match", Default {
        n3 = One Button Dialog(message="Case not matched!!") -> ()  [unwired: 1 in, 1 out]
      }
      frame "Get File Info" {
        n4 = List Folder(path=w48) -> (path out=w50:path, filenames=w51:string[])  [unwired: 3 in, 2 out]
        n5 = for {
          N -> [w104]
          tunnel: w51 -> [w123] mode=indexing
          shift-right: [w116] -> w38
          shift-left: path[] [] -> [w118]
          tunnel: w50 -> [w117]
          i -> [w105]
          n6 = Divide(x=w105, y=w104) -> (x/y=w107:dbl)
          n7 = Search/Split String(string=w123, search string/char (-)=".vec") -> (substring before match=w114:string, match + rest of string=w120:string)  [unwired: 1 in, 1 out]
          n8 = Multiply(x=w107, y=100) -> (x*y=w108:dbl)
          n9 = Concatenate Strings(w114, w120) -> (w119:string)
          n10 = String Length(string=w120) -> (length=w121:i32)
          n11 = Search/Split String(string=w114, search string/char (-)="_modified") -> (match + rest of string=w112:string)  [unwired: 1 in, 2 out]
          n12 = local write "Progress Bar"(w108) -> ()
          n13 = Greater Than 0?(x=w121) -> (x > 0?=w115:bool)
          n14 = String Length(string=w112) -> (length=w111:i32)
          n15 = Equal To 0?(x=w111) -> (x = 0?=w110:bool)
          n16 = And(x=w115, y=w110) -> (x .and. y?=w109:bool)
          n17 = case shown="True" w109 {
            tunnel: w119 -> [_ w129]
            tunnel: w118 -> [w124 w125]
            tunnel: w117 -> [_ w128]
            tunnel: [w124 w126] -> w116
            frame False {
            }
            frame True {
              n18 = Build Path(base path=w128, name or relative path=w129) -> (appended path=w127:path)
              n19 = Build Array (concatenate)(w125, w127) -> (w126:path[])
            }
          }
        }
        "File Array" <- w38
        n20 = local write "Position Array"(dbl[][] [] ("Position Array")) -> ()
        n21 = local write "Data Array"(dbl[][][] [] ("Data Array")) -> ()
        n22 = Array Size(array=w38) -> (size(s)=w42:i32)
        n23 = Reciprocal(x=w47) -> (1/x=w45:dbl)
        n24 = Multiply(x=w45, y=w42) -> (x*y=w46:dbl)
        n25 = for {
          N -> [w62]
          tunnel: w38 -> [w69] mode=indexing
          tunnel: [w58] -> w37 mode=indexing
          tunnel: [w66] -> w33 mode=indexing
          tunnel: "Collecting Raw data from all vectors" ("Status") -> [w60]
          i -> [w61]
          n26 = local write "Status"(w60) -> ()
          n27 = Divide(x=w61, y=w62) -> (x/y=w64:dbl)
          n28 = Read from Text File(file (use dialog)=w69) -> (text=w81:string)  [unwired: 3 in, 3 out]
          n29 = Multiply(x=w64, y=100) -> (x*y=w63:dbl)
          n30 = Match Pattern(string=w81, regular expression="\n") -> (after substring=w77:string)  [unwired: 1 in, 3 out]
          n31 = local write "Progress Bar"(w63) -> ()
          n32 = Spreadsheet String To Array(delimiter (Tab)=",", format string="%.6f", spreadsheet string=w77) -> (array=w55:dbl[][])  [unwired: 1 in]
          n33 = Transpose 2D Array(2D array=w55) -> (transposed array=w76:dbl[][])
          n34 = Index Array(array=w76, index (row)=4) -> (element=w73:dbl[])  [unwired: 1 in]
          n35 = call "Search_1D_Array(DBL).vi"("Array"=w73, "Element Data"=1.0) -> ("Indicies of Elements"=w59:i32[])  [unwired: 7 in]
          n36 = call "Search_1D_Array(DBL).vi"("Array"=w73, "Element Data"=-1.0) -> ("Indicies of Elements"=w70:i32[])  [unwired: 7 in]
          n37 = Build Array (concatenate)(w59, w70) -> (w71:i32[])
          n38 = Array Size(array=w71) -> (size(s)=w58:i32)
          n39 = Initialize Array(0.0 ("element"), 5 ("dimension size"), w58) -> (w67:dbl[][])
          n40 = Transpose 2D Array(2D array=w67) -> (transposed array=w68:dbl[][])
          n41 = for {
            tunnel: w55 -> [w91] mode=indexing
            shift-right: [w94] -> w66
            shift-left: w68 -> [w89]
            shift-right: [w93] -> _
            shift-left: 0 ("y") -> [w92]
            tunnel: w55 -> [w90]
            i -> [w88]
            n42 = Index Array(array=w91, index=4) -> (element=w85:dbl)
            n43 = Index Array(array=w90, index (row)=w88) -> (element=w95:dbl[])  [unwired: 1 in]
            n44 = Equal?(x=w85, y=1.0) -> (x = y?=w84:bool)
            n45 = Equal?(x=w85, y=-1.0) -> (x = y?=w83:bool)
            n46 = Or(x=w84, y=w83) -> (x .or. y?=w82:bool)
            n47 = case shown="True" w82 {
              tunnel: w95 -> [_ w101]
              tunnel: w89 -> [w98 w103]
              tunnel: [w98 w102] -> w94
              tunnel: [w97 w100] -> w93
              tunnel: w92 -> [w97 w99]
              frame False {
              }
              frame True {
                n48 = Increment(x=w99) -> (x+1=w100:i32)
                n49 = Replace Array Subset(array=w103, new element=w101, index (row)=w99) -> (w102:dbl[][])  [unwired: 1 in]
              }
            }
          }
        }
        "VectRawData(time,spot)" <- w33
        n50 = call-poly <vilib>:"Ramp Pattern.vi"("start"=0.0, "end"=w46, "samples"=w42) -> ("Ramp Pattern"=→"time s":dbl[])  [unwired: 7 in, 1 out]
        n51 = Array Max & Min(array=w37) -> (max value=→"# total vectors":i32)  [unwired: 3 out]
        "Status" <- "Getting file information from the data folder..." ("Status")
      }
      frame "Get Position" {
        n52 = local read "# total vectors"() -> (w141:i32)
        n53 = Initialize Array(T1 {"Record Length"=0.0, "CHC"=[], "u m/s"=[], "v m/s"=[], "time s"=[], "Vel mag m/s"=[], "XYZ Position"=[], " Turb Stats"=[], "Turb Stats Error"=[], "u (good)"=[], "v (good)"=[]} ("Spot Data Cluster"), w141) -> (w139:T2)
        n54 = for {
          N -> [w182]
          shift-right: [w187] -> w137
          shift-left: w139 -> [w188]
          tunnel: w130 -> [w180] mode=indexing
          tunnel: w143 -> [w189]
          tunnel: w142 -> [w181]
          tunnel: "Getting PIV spot positions for all vecotrs" ("Status") -> [w178]
          i -> [w183]
          n55 = Transpose 2D Array(2D array=w180) -> (transposed array=w179:dbl[][])
          n56 = Divide(x=w183, y=w182) -> (x/y=w185:dbl)
          n57 = Index Array(array=w179) -> (element #1=w191:dbl[], element #2=w190:dbl[])  [unwired: 4 in]
          n58 = Multiply(x=w185, y=100) -> (x*y=w186:dbl)
          n59 = for {
            tunnel: w191 -> [w198] mode=indexing
            tunnel: w190 -> [w197] mode=indexing
            tunnel: w189 -> [w196]
            shift-right: [w193] -> w187
            shift-left: w188 -> [w195]
            tunnel: w181 -> [w192]
            i -> [w194]
            n60 = in-place {
              in-place-border: w198 -> [w205]
              in-place-border: w197 -> [w204]
              in-place-border: w196 -> [w203]
              in-place-border: w192 -> [w199]
              n61 = in-place-array #1(w195, w194) -> (w202:T1)
              n62 = case shown="\"XZ\"" w199 {
                tunnel: w205 -> [w209 w215 w219]
                tunnel: w204 -> [w210 w214 w218]
                tunnel: 0.0 ("element") -> [w211 w213 w217]
                tunnel: [w208 w212 w216] -> w207
                frame "XY" {
                  n63 = Build Array(w209, w210, w211) -> (w208:dbl[])
                }
                frame "YZ" {
                  n64 = Build Array(w213, w215, w214) -> (w212:dbl[])
                }
                frame "XZ" {
                  n65 = Build Array(w219, w217, w218) -> (w216:dbl[])
                }
              }
              n66 = Add(x=w203, y=w207) -> (x+y=w201:dbl[])
              n67 = Bundle By Name(cluster=w202, "XYZ Position"=w201) -> (w200:T1)
              n68 = in-place-array #1(w200) -> (w193:T2)  [unwired: 1 out]
            }
          }
          n69 = local write "Progress Bar"(w186) -> ()
          n70 = local write "Status"(w178) -> ()
        }
        n71 = local read "# total vectors"() -> (w136:i32)
        n72 = local read "time s"() -> (w131:dbl[])
        n73 = for {
          N: w136 -> [w160]
          shift-right: [w165] -> w134
          shift-left: w137 -> [w167]
          tunnel: "Getting instantaneous data for all vectors" ("Status") -> [w164]
          tunnel: w133 -> [w151]
          tunnel: w132 -> [w157]
          tunnel: w131 -> [w149]
          tunnel: w130 -> [w166]
          i -> [w148]
          n74 = local write "Status"(w164) -> ()
          n75 = Divide(x=w148, y=w160) -> (x/y=w162:dbl)
          n76 = Index Array(array=w166, index (dim 1) #1=w148, index (dim 2) #1=2 ("disabled index (col)"), index (dim 1) #2=w148, index (dim 2) #2=3 ("disabled index (col)"), index (dim 1) #3=w148, index (dim 2) #3=4 ("disabled index (col)")) -> (element #1=w155:dbl[], element #2=w152:dbl[], element #3=w146:dbl[])  [unwired: 3 in]
          n77 = Multiply(x=w162, y=100) -> (x*y=w161:dbl)
          n78 = Negate(x=w155) -> (-x=w156:dbl[])
          n79 = Negate(x=w152) -> (-x=w153:dbl[])
          n80 = local write "Progress Bar"(w161) -> ()
          n81 = Select(t=w156, s=w157, f=w155) -> (s? t:f=w154:dbl[])
          n82 = Select(t=w153, s=w151, f=w152) -> (s? t:f=w150:dbl[])
          n83 = in-place {
            in-place-border: w154 -> [w172]
            in-place-border: w150 -> [w171]
            in-place-border: w149 -> [w169]
            in-place-border: w146 -> [w168]
            n84 = in-place-array #2(w167, w148) -> (w177:T1)
            n85 = Square(x=w172) -> (x^2=w175:dbl[])
            n86 = Square(x=w171) -> (x^2=w174:dbl[])
            n87 = Compound Arithmetic op=ADD(w175, w174) -> (w173:dbl[])
            n88 = Square Root(x=w173) -> (sqrt(x)=w170:dbl[])
            n89 = Bundle By Name(cluster=w177, "u m/s"=w172, "v m/s"=w171, "CHC"=w168, "Vel mag m/s"=w170, "time s"=w169) -> (w176:T1)
            n90 = in-place-array #2(w176) -> (w165:T2)  [unwired: 1 out]
          }
        }
      }
      frame "Process Data" {
        n91 = for {
          N -> [w238]
          tunnel: w222 -> [w236]
          tunnel: w221 -> [w235]
          tunnel: w220 -> [w234] mode=indexing
          shift-right: [w243] -> w225
          shift-left: w223 -> [w248]
          i -> [w237]
          n92 = Transpose 2D Array(2D array=w234) -> (transposed array=w233:dbl[][])
          n93 = Divide(x=w237, y=w238) -> (x/y=w240:dbl)
          n94 = Index Array(array=w233, index (row) #1=2 ("index (row)")) -> (element #1=w231:dbl[], element #2=w230:dbl[], element #3=w229:dbl[])  [unwired: 5 in]
          n95 = call "Search_1D_Array(DBL).vi"("Array"=w229, "Element Data"=1.0) -> ("Indicies of Elements"=w228:i32[])  [unwired: 7 in]
          n96 = Multiply(x=w240, y=100) -> (x*y=w241:dbl)
          n97 = Negate(x=w231) -> (-x=w247:dbl[])
          n98 = Negate(x=w230) -> (-x=w246:dbl[])
          n99 = local write "Progress Bar"(w241) -> ()
          n100 = Select(t=w247, s=w235, f=w231) -> (s? t:f=w245:dbl[])
          n101 = Select(t=w246, s=w236, f=w230) -> (s? t:f=w244:dbl[])
          n102 = for {
            tunnel: w245 -> [w253]
            tunnel: w244 -> [w252]
            tunnel: w228 -> [w249] mode=indexing
            shift-right: [w250] -> w243
            shift-left: w248 -> [w251]
            n103 = in-place {
              in-place-border: w253 -> [w262]
              in-place-border: w252 -> [w261]
              in-place-border: w249 -> [w254]
              n104 = in-place-array #3(w251, w249) -> (w256:T1)
              n105 = Unbundle By Name(w256) -> ("Record Length"=w257:dbl)
              n106 = Index Array(array=w262, index=w254) -> (element=w259:dbl)
              n107 = Index Array(array=w261, index=w254) -> (element=w258:dbl)
              n108 = Equal To 0?(x=w257) -> (x = 0?=w260:bool)
              n109 = case shown="False" w260 {
                tunnel: [w270 w275] -> w255
                tunnel: w258 -> [w265 w272]
                tunnel: w256 -> [w271 w274]
                tunnel: w259 -> [w266 w273]
                frame True {
                  # "Initialise Spot Data Cluster"
                  n110 = Build Array(w265) -> (w263:dbl[])
                  n111 = Build Array(w266) -> (w264:dbl[])
                  n112 = call "Generic_Weighted_Stats.vi"("v"=w263, "u"=w264) -> ("Turbulence Statistics"=w268:T3)  [unwired: 9 in]
                  n113 = Build Array(w268) -> (w267:T4)
                  n114 = Bundle By Name(cluster=w271, "Record Length"=1.0, "Turb Stats"=w267, "Turb Stats Error"=w267, "u (good)"=w264, "v (good)"=w263) -> (w270:T1)
                }
                frame False {
                  n115 = in-place {
                    in-place-border: w273 -> [w281]
                    in-place-border: w272 -> [w280]
                    n116 = in-place-cluster #4(w274) -> ("Record Length"=w292:dbl, "Turb Stats"=w294:T4, "Turb Stats Error"=w284:T4, "u (good)"=w282:dbl[], "v (good)"=w279:dbl[])
                    n117 = Insert Into Array(array=w282, new element=w281) -> (w277:dbl[])  [unwired: 1 in]
                    n118 = Insert Into Array(array=w279, new element=w280) -> (w278:dbl[])  [unwired: 1 in]
                    n119 = call "Generic_Weighted_Stats.vi"("v"=w278, "u"=w277) -> ("Turbulence Statistics"=w283:T3)  [unwired: 9 in]
                    n120 = Insert Into Array(array=w294, new element=w283) -> (w293:T4)  [unwired: 1 in]
                    n121 = Decrement(x=w292) -> (x-1=w291:dbl)
                    n122 = Index Array(array=w293, index=w291) -> (element=w290:T3)
                    n123 = Divide(x=w290, y=w283) -> (x/y=w289:T3)
                    n124 = Subtract(x=w289, y=1.0 ("Record Length")) -> (x-y=w287:T3)
                    n125 = Increment(x=w292) -> (x+1=w285:dbl)
                    n126 = Absolute Value(x=w287) -> (abs(x)=w276:T3)
                    n127 = Insert Into Array(array=w284, new element=w276) -> (w286:T4)  [unwired: 1 in]
                    n128 = in-place-cluster #4("Record Length"=w285, "Turb Stats"=w293, "Turb Stats Error"=w286, "u (good)"=w277, "v (good)"=w278) -> (w275:T1)
                  }
                }
              }
              n129 = in-place-array #3(w255) -> (w250:T2)  [unwired: 1 out]
            }
          }
        }
        n130 = local write "Status"("Calculating turbulent statistics for only good vectors" ("Status")) -> ()
      }
      frame "Adjust Record Lengths" {
        n131 = for {
          N -> [w310]
          tunnel: w306 -> [w314] mode=indexing
          tunnel: [w312] -> w305 mode=indexing
          tunnel: [w313] -> w302 mode=indexing
          tunnel: [w311] -> w299 mode=indexing
          tunnel: [w310] -> w295
          n132 = Unbundle By Name(w314) -> ("Record Length"=w312:dbl, "time s"=w313:dbl[])
          n133 = Equal To 0?(x=w312) -> (x = 0?=w311:bool)
        }
        n134 = Boolean To (0,1)(Boolean=w299) -> (0, 1=w298:i16[])
        n135 = Array Max & Min(array=w305) -> (max value=w304:dbl)  [unwired: 3 out]
        n136 = Array Max & Min(array=w302) -> (max value=→"Tmax":dbl)  [unwired: 3 out]
        n137 = Add Array Elements(numeric array=w298) -> (sum=→"# vectors without records":i16)
        n138 = To Long Integer(number=w304) -> (32bit integer=→"Max Record Length":i32)
        n139 = local write "Status"("Adjusting the record lengths of each spot..." ("Status")) -> ()
        n140 = for {
          N: w295 -> [w320]
          tunnel: w304 -> [w322]
          shift-right: [w316] -> w307
          shift-left: w306 -> [w317]
          i -> [w315]
          n141 = in-place {
            in-place-border: w322 -> [w325]
            n142 = in-place-array #5(w317, w315) -> (w324:T1)
            n143 = in-place {
              in-place-border: w325 -> [w326]
              n144 = in-place-cluster #6(w324) -> ("Record Length"=w327:dbl, "Turb Stats Error"=w330:T4, "Turb Stats"=w328:T4)
              n145 = Subtract(x=w326, y=w327) -> (x-y=w333:dbl)
              n146 = Greater Than 0?(x=w333) -> (x > 0?=w334:bool)
              n147 = case shown="True" w334 {
                tunnel: w333 -> [_ w344]
                tunnel: [w335 w338] -> w332
                tunnel: [w337 w341] -> w331
                tunnel: w330 -> [w337 w343]
                tunnel: [w336 w340] -> w329
                tunnel: w328 -> [w336 w342]
                tunnel: w327 -> [w335 w338]
                frame False {
                }
                frame True {
                  n148 = To Long Integer(number=w344) -> (32bit integer=w339:i32)
                  n149 = for {
                    N: w339 -> [_]
                    shift-right: [w350] -> w341
                    shift-left: w343 -> [w351]
                    shift-right: [w349] -> w340
                    shift-left: w342 -> [w348]
                    w345 = 1 ("n")
                    n150 = Rotate 1D Array(1:w351, 2:w345) -> (0:w352:T4)
                    n151 = Rotate 1D Array(1:w348, 2:w345) -> (0:w347:T4)
                    n152 = Index Array(array=w352) -> (element=w353:T3)  [unwired: 1 in]
                    n153 = Index Array(array=w347) -> (element=w346:T3)  [unwired: 1 in]
                    n154 = Insert Into Array(array=w351, new element=w353) -> (w350:T4)  [unwired: 1 in]
                    n155 = Insert Into Array(array=w348, new element=w346) -> (w349:T4)  [unwired: 1 in]
                  }
                }
              }
              n156 = in-place-cluster #6("Record Length"=w332, "Turb Stats Error"=w331, "Turb Stats"=w329) -> (w323:T1)
            }
            n157 = in-place-array #5(w323) -> (w316:T2)  [unwired: 1 out]
          }
          n158 = Divide(x=w315, y=w320) -> (x/y=w319:dbl)
          n159 = Multiply(x=w319, y=100) -> (x*y=w321:dbl)
          n160 = local write "Progress Bar"(w321) -> ()
        }
      }
      frame "Create Files" {
        n161 = Index Array(array=w370) -> (element=w384:T1)  [unwired: 1 in]
        n162 = Equal?(x=w365, y=1) -> (x = y?=w360:bool)
        n163 = Build Path(base path=w386, name or relative path=w387) -> (appended path=w363:path)
        n164 = call "Get Cluster Element Names.vi"("Cluster"=w384) -> ("Element Names"=w383:string[])  [unwired: 9 in, 1 out]
        n165 = Unbundle By Name(w384) -> ("Turb Stats"=w374:T4)
        n166 = call <vilib>:"Check if File or Folder Exists.vi"("path"=w363) -> ("file or folder exists?"=w361:bool, "dup path"=w362:path)  [unwired: 8 in, 1 out]
        n167 = And(x=w360, y=w361) -> (x .and. y?=w356:bool)
        n168 = case shown="True" w356 {
          tunnel: [w391 path "" ("dup path")] -> w359
          tunnel: w362 -> [w391 _]
          frame False {
          }
          frame True {
            w394 = T5 1 items=["no dialog", "OK message", "continue or stop message", "OK message + warnings", "continue/stop + warnings"] ("type of dialog (OK msg:1)")
            n169 = call <vilib>:"Simple Error Handler.vi"("type of dialog (OK msg:1)"=w394, "error in (no error)"=errorcluster {"status"=TRUE, "code"=0, "source"="Folder already exists, please select a new case name or results folder"}) -> ()  [unwired: 3 in, 5 out]
          }
        }
        n170 = Delete From Array(array=w383, length=5, index=6) -> (deleted portion=w369:string[], array with subset deleted=w379:string[])
        n171 = Index Array(array=w374) -> (element=w373:T3)  [unwired: 1 in]
        n172 = call "Get Cluster Element Names.vi"("Cluster"=w373) -> ("Element Names"=w380:string[])  [unwired: 9 in, 1 out]
        n173 = Delete From Array(array=w369, length=1, index=0) -> (array with subset deleted=w368:string[])  [unwired: 1 out]
        n174 = for {
          tunnel: w368 -> [w397] mode=indexing
          tunnel: w380 -> [w396]
          tunnel: [w395] -> w378 mode=indexing
          n175 = for {
            tunnel: w397 -> [w401]
            tunnel: w396 -> [w399] mode=indexing
            tunnel: [w398] -> w395 mode=indexing
            n176 = Concatenate Strings(w401, "_" ("string"), w399) -> (w398:string)
          }
        }
        n177 = Index Array(array=w378) -> (element #1=w377:string[], element #2=w376:string[])  [unwired: 4 in]
        n178 = Build Array (concatenate)(w379, w377, w376) -> (w375:string[])
        n179 = for {
          tunnel: w375 -> [w404] mode=indexing
          tunnel: [w406] -> w372 mode=indexing
          w410 = "_" ("Replace with")
          n180 = call <vilib>:"Trim Whitespace.vi"("string"=w404) -> ("trimmed string"=w402:string)  [unwired: 1 in]
          n181 = call "Replace_Character.vi"("Replace with"="_", "Input String"=w402, "Search For"=" ") -> ("Output string"=w405:string)  [unwired: 1 out]
          n182 = call "Replace_Character.vi"("Replace with"=w410, "Input String"=w405, "Search For"="(") -> ("Output string"=w412:string)  [unwired: 1 out]
          n183 = call "Replace_Character.vi"("Replace with"=w410, "Input String"=w412, "Search For"=")") -> ("Output string"=w409:string)  [unwired: 1 out]
          n184 = call "Replace_Character.vi"("Replace with"="", "Input String"=w409, "Search For"="/") -> ("Output string"=w406:string)  [unwired: 1 out]
        }
        "Variable Names" <- w372
        n185 = Build Path(base path=w359, name or relative path="ENSI_all.case") -> (appended path=→"ALL filepath":path)
        n186 = local read "Max Record Length"() -> (w371:i32)
        n187 = for {
          N: w371 -> [_]
          tunnel: w359 -> [w432]
          tunnel: w372 -> [w431]
          tunnel: [w430] -> w390 mode=indexing
          i -> [w426]
          n188 = Number To Decimal String(number=w426, width (-)=i16 4) -> (decimal integer string=w424:string)
          n189 = call "Whitespace_to_Zeros.vi"("Input String"=w424) -> ("Output String"=w420:string)  [unwired: 6 in]
          n190 = Concatenate Strings("ENSI_" ("name or relative path"), w420) -> (w416:string)
          n191 = Concatenate Strings(w416, ".var" ("name or relative path")) -> (w415:string)
          n192 = for {
            tunnel: w432 -> [w439]
            tunnel: [w434] -> w427 mode=indexing
            tunnel: w431 -> [_] mode=indexing
            tunnel: w415 -> [w433]
            i -> [w438]
            n193 = Increment(x=w438) -> (x+1=w437:i32)
            n194 = Number To Decimal String(number=w437) -> (decimal integer string=w436:string)  [unwired: 1 in]
            n195 = Concatenate Strings(w433, w436) -> (w435:string)
            n196 = Build Path(base path=w439, name or relative path=w435) -> (appended path=w434:path)
          }
          n197 = Concatenate Strings(w416, ".case" ("name or relative path")) -> (w423:string)
          n198 = Concatenate Strings(w416, ".geo" ("name or relative path")) -> (w419:string)
          n199 = Build Path(base path=w432, name or relative path=w423) -> (appended path=w428:path)
          n200 = Build Path(base path=w432, name or relative path=w419) -> (appended path=w429:path)
          n201 = Build Array (concatenate)(w428, w429, w427) -> (w430:path[])
        }
        "File Paths" <- w390
        n202 = Select(t="End Time", s=w356, f="Setup Files" ("t")) -> (s? t:f=w358:string)
      }
      frame "Setup Files" {
        n203 = local read "File Paths"() -> (w445:path[][])
        n204 = local write "Status"("Setting up case files ready to write to..." ("Status")) -> ()
        n205 = for {
          N -> [w448]
          tunnel: w445 -> [w454] mode=indexing
          i -> [w447]
          n206 = Divide(x=w447, y=w448) -> (x/y=w446:dbl)
          n207 = Number To Decimal String(number=w447, width (-)=i16 4) -> (decimal integer string=w452:string)
          n208 = call "Whitespace_to_Zeros.vi"("Input String"=w452) -> ("Output String"=w451:string)  [unwired: 6 in]
          n209 = Multiply(x=w446, y=100) -> (x*y=w450:dbl)
          n210 = for {
            tunnel: w454 -> [w457] mode=indexing
            tunnel: w451 -> [w455]
            i -> [w456]
            n211 = case shown="2, Default" w456 {
              tunnel: w457 -> [w468 w493 w512]
              tunnel: w456 -> [_ _ w507]
              tunnel: w455 -> [w458 _ _]
              frame 0 {
                n212 = local read "Variable Names"() -> (w472:string[])
                n213 = for {
                  tunnel: w472 -> [w484] mode=indexing
                  tunnel: [w482] -> w467 mode=indexing
                  tunnel: w458 -> [w479]
                  i -> [w486]
                  n214 = Increment(x=w486) -> (x+1=w487:i32)
                  n215 = Concatenate Strings(" ENSI_", w479, ".var") -> (w481:string)
                  n216 = Number To Decimal String(number=w487) -> (decimal integer string=w485:string)  [unwired: 1 in]
                  n217 = Concatenate Strings(w481, w485) -> (w483:string)
                  n218 = Concatenate Strings("scalar per node: ", w484, w483) -> (w482:string)
                }
                n219 = Concatenate Strings("model: ENSI_", w458, ".geo") -> (w460:string)
                n220 = Build Array (concatenate)("FORMAT", "type: ensight gold", "GEOMETRY", w460, "VARIABLE", w467) -> (w466:string[])
                n221 = for {
                  tunnel: w466 -> [w477] mode=indexing
                  shift-right: [w475] -> w470
                  shift-left: "" -> [w473]
                  n222 = Concatenate Strings(w477, "\r\n") -> (w474:string)
                  n223 = Concatenate Strings(w473, w474) -> (w475:string)
                }
                n224 = call "Write_File_Simple.vi"("append to file? (new file:F)"=FALSE, "character string"=w470, "file path"=w468) -> ()  [unwired: 2 out]
              }
              frame 1 {
                n225 = local read "# total vectors"() -> (w491:i32)
                n226 = Number To Decimal String(number=w491) -> (decimal integer string=w490:string)  [unwired: 1 in]
                n227 = Build Array (concatenate)(string[] ["EnSight Model Geometry File", "EnSight 9.2 ", "node id assign", "element id assign", "part", "         1", "Point field", "coordinates"], w490) -> (w489:string[])
                n228 = for {
                  tunnel: w489 -> [w501] mode=indexing
                  shift-right: [w499] -> w495
                  shift-left: "" -> [w497]
                  n229 = Concatenate Strings(w501, "\r\n") -> (w498:string)
                  n230 = Concatenate Strings(w497, w498) -> (w499:string)
                }
                n231 = call "Write_File_Simple.vi"("append to file? (new file:F)"=FALSE, "character string"=w495, "file path"=w493) -> ()  [unwired: 2 out]
              }
              frame 2, Default {
                n232 = local read "Variable Names"() -> (w508:string[])
                n233 = Subtract(x=w507, y=2) -> (x-y=w505:i32)
                n234 = Index Array(array=w508, index=w505) -> (element=w504:string)
                n235 = Build Array (concatenate)(w504, string[] ["part", "         1", "coordinates"]) -> (w502:string[])
                n236 = for {
                  tunnel: w502 -> [w517] mode=indexing
                  shift-right: [w515] -> w510
                  shift-left: "" -> [w513]
                  n237 = Concatenate Strings(w517, "\r\n") -> (w514:string)
                  n238 = Concatenate Strings(w513, w514) -> (w515:string)
                }
                n239 = call "Write_File_Simple.vi"("append to file? (new file:F)"=FALSE, "character string"=w510, "file path"=w512) -> ()  [unwired: 2 out]
              }
            }
          }
          n240 = local write "Progress Bar"(w450) -> ()
        }
      }
      frame "Collect Data" {
        w519 = T2 []  # Array
        n241 = local read "Max Record Length"() -> (w525:i32)
        n242 = local read "ALL filepath"() -> (w526:path)
        n243 = local write "Status"("Gathering all the data ready to write to file..." ("Status")) -> ()
        n244 = Number To Decimal String(number=w525) -> (decimal integer string=w529:string)  [unwired: 1 in]
        n245 = for {
          N -> [w532]
          tunnel: w524 -> [w547] mode=indexing
          tunnel: [w538] -> w523 mode=indexing
          tunnel: [w537] -> w522 mode=indexing
          i -> [w533]
          n246 = Unbundle By Name(w547) -> ("Record Length"=w546:dbl, "CHC"=w545:dbl[], "u m/s"=w544:dbl[], "v m/s"=w543:dbl[], "time s"=w542:dbl[], "Vel mag m/s"=w541:dbl[], "Turb Stats"=w540:T4, "Turb Stats Error"=w539:T4, "XYZ Position"=w537:dbl[])
          n247 = Divide(x=w533, y=w532) -> (x/y=w535:dbl)
          n248 = Multiply(x=w535, y=100) -> (x*y=w536:dbl)
          n249 = local write "Progress Bar"(w536) -> ()
          n250 = for {
            tunnel: w546 -> [w558]
            tunnel: w545 -> [w557] mode=indexing
            tunnel: w544 -> [w556] mode=indexing
            tunnel: w543 -> [w555] mode=indexing
            tunnel: w542 -> [w554] mode=indexing
            tunnel: w541 -> [w553] mode=indexing
            tunnel: w540 -> [w552] mode=indexing
            tunnel: w539 -> [w550] mode=indexing
            tunnel: [w548] -> w538 mode=indexing
            n251 = Cluster To Array(cluster=w552) -> (array=w551:dbl[])
            n252 = Cluster To Array(cluster=w550) -> (array=w549:dbl[])
            n253 = Build Array (concatenate)(w558, w557, w556, w555, w554, w553, w551, w549) -> (w548:dbl[])
          }
        }
        "Data Array" <- w523
        n254 = call <vilib>:"Check if File or Folder Exists.vi"("path"=w526) -> ("file or folder exists?"=w527:bool, "dup path"=w528:path)  [unwired: 8 in, 1 out]
        n255 = case shown="False" w527 {
          tunnel: w528 -> [w583 _]
          tunnel: w529 -> [w568 _]
          tunnel: w525 -> [w561 _]
          frame False {
            n256 = local read "Tmax"() -> (w559:dbl)
            n257 = local read "Variable Names"() -> (w575:string[])
            n258 = call-poly <vilib>:"Ramp Pattern.vi"("end"=w559, "samples"=w561) -> ("Ramp Pattern"=w560:dbl[])  [unwired: 8 in, 1 out]
            n259 = for {
              tunnel: w575 -> [w592] mode=indexing
              tunnel: [w590] -> w574 mode=indexing
              i -> [w594]
              n260 = Increment(x=w594) -> (x+1=w595:i32)
              n261 = Number To Decimal String(number=w595) -> (decimal integer string=w593:string)  [unwired: 1 in]
              n262 = Concatenate Strings(" ENSI_****.var", w593) -> (w591:string)
              n263 = Concatenate Strings("scalar per node: ", w592, w591) -> (w590:string)
            }
            n264 = Concatenate Strings("number of steps: ", w568) -> (w566:string)
            n265 = Number To Fractional String(number=w560, precision (6)=i16 1) -> (F-format string=w562:string[])  [unwired: 2 in]
            n266 = Build Array (concatenate)("FORMAT", "type: ensight gold", "GEOMETRY", "model: ENSI_****.geo", "VARIABLE", w574, "TIME", "time set: 1", w566, "filename start number: 000", "filename increment: 0001", "time values:", w562) -> (w571:string[])
            n267 = for {
              tunnel: w571 -> [w588] mode=indexing
              shift-right: [w586] -> w572
              shift-left: "" -> [w584]
              n268 = Concatenate Strings(w588, "\r\n") -> (w585:string)
              n269 = Concatenate Strings(w584, w585) -> (w586:string)
            }
            n270 = call "Write_File_Simple.vi"("append to file? (new file:F)"=FALSE, "character string"=w572, "file path"=w583) -> ()  [unwired: 2 out]
          }
          frame True {
          }
        }
        n271 = Transpose 2D Array(2D array=w522) -> (transposed array=→"Position Array":dbl[][])
      }
      frame "Save Data" {
        n272 = local read "Position Array"() -> (w599:dbl[][])
        n273 = local read "Data Array"() -> (w600:dbl[][][])
        n274 = local read "File Paths"() -> (w601:path[][])
        n275 = for {
          N -> [w606]
          tunnel: w601 -> [w612] mode=indexing
          tunnel: w600 -> [w611]
          tunnel: w599 -> [w610]
          i -> [w605]
          # "Loop Time"
          n276 = Divide(x=w605, y=w606) -> (x/y=w608:dbl)
          n277 = Multiply(x=w608, y=100) -> (x*y=w609:dbl)
          n278 = local write "Progress Bar"(w609) -> ()
          n279 = for {
            tunnel: w612 -> [w617] mode=indexing
            tunnel: w611 -> [w616]
            tunnel: w605 -> [w615]
            tunnel: w610 -> [w613]
            i -> [w614]
            # "Loop Variable"
            n280 = case shown="1" w614 {
              tunnel: w617 -> [_ w623 w634]
              tunnel: w614 -> [_ _ w643]
              tunnel: w616 -> [_ _ w640]
              tunnel: w615 -> [_ _ w638]
              tunnel: w613 -> [_ w622 _]
              frame 0 {
              }
              frame 1 {
                n281 = Index Array(array=w622) -> (element #1=w621:dbl[], element #2=w620:dbl[], element #3=w619:dbl[])  [unwired: 6 in]
                n282 = Build Array (concatenate)(w621, w620, w619) -> (w618:dbl[])
                n283 = for {
                  tunnel: w618 -> [w627] mode=indexing
                  shift-right: [w633] -> w624
                  shift-left: "" -> [w632]
                  w628 = T5 4 items=["no dialog", "OK message", "continue or stop message", "OK message + warnings", "continue/stop + warnings"] ("type of dialog (OK msg:1)")
                  n284 = call "Ensight_Format_Check.vi"("Input Number"=w627) -> ("error"=w630:errorcluster, "Output string"=w631:string)  [unwired: 8 in, 1 out]
                  n285 = Concatenate Strings(w632, w631) -> (w633:string)
                  n286 = call <vilib>:"Simple Error Handler.vi"("error source (\" \")"="GEOM" ("error source (\" \")"), "type of dialog (OK msg:1)"=w628, "error in (no error)"=w630) -> ()  [unwired: 2 in, 5 out]
                }
                n287 = call "Write_File_Simple.vi"("append to file? (new file:F)"=TRUE, "character string"=w624, "file path"=w623) -> ()  [unwired: 2 out]
              }
              frame 2, Default {
                n288 = Subtract(x=w643, y=2) -> (x-y=w639:i32)
                n289 = Index Array(array=w640, index (dim 1)=w638, index (dim 2)=w639) -> (element=w637:dbl[])  [unwired: 1 in]
                n290 = for {
                  tunnel: w637 -> [w644] mode=indexing
                  shift-right: [w653] -> w635
                  shift-left: "" -> [w652]
                  tunnel: w634 -> [w649]
                  w645 = T5 4 items=["no dialog", "OK message", "continue or stop message", "OK message + warnings", "continue/stop + warnings"] ("type of dialog (OK msg:1)")
                  n291 = Path To String(path=w649) -> (string=w648:string)
                  n292 = call "Ensight_Format_Check.vi"("Input Number"=w644) -> ("error"=w650:errorcluster, "Output string"=w651:string)  [unwired: 8 in, 1 out]
                  n293 = Concatenate Strings("VAR file: " ("error source (\" \")"), w648) -> (w646:string)
                  n294 = call <vilib>:"Simple Error Handler.vi"("error source (\" \")"=w646, "type of dialog (OK msg:1)"=w645, "error in (no error)"=w650) -> ()  [unwired: 2 in, 5 out]
                  n295 = Concatenate Strings(w652, w651) -> (w653:string)
                }
                n296 = call "Write_File_Simple.vi"("append to file? (new file:F)"=TRUE, "character string"=w635, "file path"=w634) -> ()  [unwired: 2 out]
              }
            }
          }
        }
        n297 = local write "Status"("Wrting the data to file..." ("Status")) -> ()
      }
      frame "End Time" {
        n298 = local write "Position Array"(dbl[][] [] ("Position Array")) -> ()
        n299 = local write "Data Array"(dbl[][][] [] ("Data Array")) -> ()
      }
    }
  }
  "Progress Bar" <- u8 0 ("Progress Bar")
